vi "Oxford-1820-Main.v.vi"() -> ()   [LabVIEW 2013, in "Mercury iXX.lvlib"]
uses:
  <instrlib>/Mercury iXX/Mercury iXX.lvlib
  <instrlib>/Mercury iXX/Public/Controls/Unit String.ctl
  <instrlib>/Mercury iXX/Public/Libraries/Temperature/Controls/Temperature Device (Read).ctl
  <instrlib>/Mercury iXX/Public/Controls/Manufacturing Data.ctl
  <instrlib>/Mercury iXX/Public/Libraries/Temperature/Controls/Temperature Sensor Type.ctl
  <instrlib>/Mercury iXX/Public/Libraries/Temperature/Controls/Excitation Cluster.ctl
  <instrlib>/Mercury iXX/Public/Libraries/Temperature/Controls/Excitation Type.ctl
  <instrlib>/Mercury iXX/Public/Libraries/Temperature/Controls/Calibration Cluster.ctl
  <instrlib>/Mercury iXX/Public/Libraries/Temperature/Controls/Calibration Interpolation.ctl
  <instrlib>/Mercury iXX/Public/Libraries/Temperature/Controls/Loop Cluster.ctl
  <instrlib>/Mercury iXX/Public/Libraries/Temperature/Controls/Temperature Signals Cluster.ctl
  <instrlib>/Mercury iXX/Public/Libraries/Heater/Controls/Heater Device (Read).ctl
  <instrlib>/Mercury iXX/Public/Libraries/Heater/Controls/Heater Signals Cluster.ctl
  <instrlib>/Mercury iXX/Public/Libraries/Level Meter/Controls/Level Meter (Read).ctl
  <instrlib>/Mercury iXX/Public/Libraries/Level Meter/Controls/Nitrogen Configuration.ctl
  <instrlib>/Mercury iXX/Public/Libraries/Level Meter/Controls/Frequency Configuration.ctl
  <instrlib>/Mercury iXX/Public/Libraries/Level Meter/Controls/Signals.ctl
  <instrlib>/Mercury iXX/Public/Libraries/Level Meter/Controls/Helium Configuration.ctl
  <instrlib>/Mercury iXX/Public/Libraries/Level Meter/Controls/Resistance Configuration.ctl
  <instrlib>/Mercury iXX/Public/Libraries/Level Meter/Controls/Pre-Pulse.ctl
  <instrlib>/Mercury iXX/Public/Libraries/Level Meter/Controls/Pulse.ctl
  <instrlib>/Mercury iXX/Public/Libraries/Auxiliary/Controls/AUX Device (Read).ctl
  <instrlib>/Mercury iXX/Public/Libraries/Auxiliary/Controls/AUX Signals (Read).ctl
  <instrlib>/Mercury iXX/Public/Libraries/Magnet/Controls/Device (Read).ctl
  <instrlib>/Mercury iXX/Public/Libraries/Magnet/Controls/Signals (Read).ctl
  <instrlib>/Mercury iXX/Public/Libraries/Magnet/Controls/Identifier.ctl
  <instrlib>/Mercury iXX/Public/Libraries/Pressure/Controls/Pressure Device (Read).ctl
  <instrlib>/Mercury iXX/Public/Libraries/Pressure/Controls/Pressure Sensor Type.ctl
  <instrlib>/Mercury iXX/Public/Libraries/Pressure/Controls/Calibration Cluster.ctl
  <instrlib>/Mercury iXX/Public/Libraries/Pressure/Controls/Calibration Interpolation.ctl
  <instrlib>/Mercury iXX/Public/Libraries/Pressure/Controls/Loop Cluster.ctl
  <instrlib>/Mercury iXX/Public/Libraries/Pressure/Controls/Pressure Signals Cluster.ctl
  <instrlib>/Mercury iXX/Public/Libraries/Magnet/Controls/PSU Actions.ctl
  <instrlib>/Mercury iXX/Public/Libraries/Magnet/Controls/Switch Heater.ctl
  <instrlib>/Mercury iXX/Public/Controls/Comms Transport Layer.ctl
  <instrlib>/Mercury iXX/Private/Controls/Query Dynamic Reference.ctl
  <instrlib>/Mercury iXX/Public/Controls/Mercury Reference.ctl
  <instrlib>/Mercury iXX/Public/Libraries/Magnet/Open/Open Magnet Device.vi
  <instrlib>/Mercury iXX/Public/Libraries/Magnet/Configuration/Set/PSU Action Status (Set).vi
  <instrlib>/Mercury iXX/Public/Libraries/Magnet/Signals/Read/Current (Read).vi
  <instrlib>/Mercury iXX/Public/Libraries/Magnet/Signals/Read/Persistant Current (Read).vi
  <instrlib>/Mercury iXX/Public/Libraries/Magnet/Signals/Read/Switch Heater Status (Read).vi
  <instrlib>/Mercury iXX/Public/Libraries/Magnet/Signals/Set/Switch Heater No Check (Set).vi
  <instrlib>/Mercury iXX/Public/Libraries/System/Read/Time (Read).vi
  <instrlib>/Mercury iXX/Public/Libraries/Magnet/Signals/Set/Target Field Rate (Set).vi
  <instrlib>/Mercury iXX/Public/Libraries/Magnet/Signals/Set/Target Field (Set).vi
  <instrlib>/Mercury iXX/Public/Libraries/System/Open/Open Device.vi
  <instrlib>/Mercury iXX/Public/Libraries/Control Loop/Configuration/Set/Sweep Mode (Set).vi
  <instrlib>/Mercury iXX/Public/Libraries/System/Open/Open System.vi
  <instrlib>/Mercury iXX/Public/Libraries/System/Read/Catalogue (Read).vi
  <instrlib>/Mercury iXX/Public/Libraries/System/Read/Display Automatic Dimming (Read).vi
  <instrlib>/Mercury iXX/Public/Libraries/System/Read/Display Automatic Dimming Time (Read).vi
  <instrlib>/Mercury iXX/Public/Libraries/System/Read/Display Brightness (Read).vi
  <instrlib>/Mercury iXX/Public/Libraries/System/Read/Date (Read).vi
  <instrlib>/Mercury iXX/Public/Libraries/System/Read/DateTime (Read).vi
  <instrlib>/Mercury iXX/Public/Libraries/System/Read/HVer (Read).vi
  <instrlib>/Mercury iXX/Public/Libraries/System/Read/FVer (Read).vi
  <instrlib>/Mercury iXX/Public/Libraries/System/Read/Serial Number (Read).vi
  <instrlib>/Mercury iXX/Public/Libraries/System/Read/Flash Space (Read).vi
  <instrlib>/Mercury iXX/Public/Libraries/System/Read/Mode (Read).vi
  <instrlib>/Mercury iXX/Public/Libraries/System/Set/DateTime (Set).vi
  <instrlib>/Mercury iXX/Public/Libraries/Temperature/Open/Open Temperature Device.vi
  <instrlib>/Mercury iXX/Public/Libraries/Temperature/Configuration/Read/Serial Number (Read).vi
  <instrlib>/Mercury iXX/Public/Libraries/Temperature/Configuration/Read/Nickname (Read).vi
  <instrlib>/Mercury iXX/Public/Libraries/Temperature/Configuration/Read/Excitation Magnitude (Read).vi
  <instrlib>/Mercury iXX/Public/Libraries/Temperature/Configuration/Read/Temperature Sensor (Read).vi
  <instrlib>/Mercury iXX/Public/Libraries/Temperature/Configuration/Read/Excitation Type (Read).vi
  <instrlib>/Mercury iXX/Public/Libraries/Temperature/Configuration/Read/Calibration Hot Limit (Read).vi
  <instrlib>/Mercury iXX/Public/Libraries/Temperature/Configuration/Read/Calibration Cold Limit (Read).vi
  <instrlib>/Mercury iXX/Public/Libraries/Temperature/Signals/Read/Voltage (Read).vi
  <instrlib>/Mercury iXX/Public/Libraries/Temperature/Signals/Read/Temperature (Read).vi
  <instrlib>/Mercury iXX/Public/Libraries/Temperature/Configuration/Read/Temperature Device (Read).vi
  <instrlib>/Mercury iXX/Public/Libraries/Control Loop/Configuration/Read/Control Loop (Read).vi
  <instrlib>/Mercury iXX/Public/Libraries/Heater/Open/Open Heater Device.vi
  <instrlib>/Mercury iXX/Public/Libraries/Heater/Configuration/Read/Heater Device (Read).vi
  <instrlib>/Mercury iXX/Public/Libraries/Heater/Configuration/Read/Nickname (Read).vi
  <instrlib>/Mercury iXX/Public/Libraries/Heater/Configuration/Read/Serial Number (Read).vi
  <instrlib>/Mercury iXX/Public/Libraries/Heater/Configuration/Read/Voltage Limit (Read).vi
  <instrlib>/Mercury iXX/Public/Libraries/Heater/Configuration/Read/Nominal Resistance (Read).vi
  <instrlib>/Mercury iXX/Public/Libraries/Heater/Configuration/Read/Maximum Power (Read).vi
  <instrlib>/Mercury iXX/Public/Libraries/Heater/Signals/Read/Voltage (Read).vi
  <instrlib>/Mercury iXX/Public/Libraries/Heater/Signals/Read/Power (Read).vi
  <instrlib>/Mercury iXX/Public/Libraries/Heater/Signals/Read/Current (Read).vi
  <instrlib>/Mercury iXX/Public/Libraries/Auxiliary/Open/Open Auxiliary Device.vi
  <instrlib>/Mercury iXX/Public/Libraries/Auxiliary/Configuration/Read/Aux Device (Read).vi
  <instrlib>/Mercury iXX/Public/Libraries/Auxiliary/Configuration/Read/Serial Number (Read).vi
  <instrlib>/Mercury iXX/Public/Libraries/Auxiliary/Configuration/Read/Minimum Gas Flow (Read).vi
  <instrlib>/Mercury iXX/Public/Libraries/Auxiliary/Configuration/Read/Gas Flow Scaling (Read).vi
  <instrlib>/Mercury iXX/Public/Libraries/Auxiliary/Configuration/Read/Temperature Error Sensitivity (Read).vi
  <instrlib>/Mercury iXX/Public/Libraries/Auxiliary/Configuration/Read/Temperature Error Voltage Sensitivity (Read).vi
  <instrlib>/Mercury iXX/Public/Libraries/Auxiliary/Configuration/Read/Valve Gearing (Read).vi
  <instrlib>/Mercury iXX/Public/Libraries/Auxiliary/Configuration/Read/Stepper Speed (Read).vi
  <instrlib>/Mercury iXX/Public/Libraries/Auxiliary/Signals/Read/Position (Read).vi
  <instrlib>/Mercury iXX/Public/Libraries/Auxiliary/Signals/Read/Percent Open (Read).vi
  <instrlib>/Mercury iXX/Public/Libraries/Pressure/Open/Open Pressure Device.vi
  <instrlib>/Mercury iXX/Public/Libraries/Pressure/Configuration/Read/Pressure Device (Read).vi
  <instrlib>/Mercury iXX/Public/Libraries/Pressure/Configuration/Read/Nickname (Read).vi
  <instrlib>/Mercury iXX/Public/Libraries/Pressure/Signals/Read/Current (Read).vi
  <instrlib>/Mercury iXX/Public/Libraries/Pressure/Signals/Read/Voltage (Read).vi
  <instrlib>/Mercury iXX/Public/Libraries/Level Meter/Open/Open Level Meter Device.vi
  <instrlib>/Mercury iXX/Public/Libraries/Level Meter/Configuration/Read/Level Meter Device (Read).vi
  <instrlib>/Mercury iXX/Public/Libraries/Level Meter/Configuration/Read/Serial Number (Read).vi
  <instrlib>/Mercury iXX/Public/Libraries/Level Meter/Configuration/Read/Helium Probe Resistance (Read).vi
  <instrlib>/Mercury iXX/Public/Libraries/Level Meter/Configuration/Read/Helium Pulse Mag (Read).vi
  <instrlib>/Mercury iXX/Public/Libraries/Level Meter/Configuration/Read/Helium Pulse Duration (Read).vi
  <instrlib>/Mercury iXX/Public/Libraries/Level Meter/Configuration/Read/Nitrogen Freq at 100 (Read).vi
  <instrlib>/Mercury iXX/Public/Libraries/Level Meter/Configuration/Read/Nitrogen Pulse Count Period (Read).vi
  <instrlib>/Mercury iXX/Public/Libraries/Level Meter/Signals/Read/Probe Resistance Helium (Read).vi
  <instrlib>/Mercury iXX/Public/Libraries/Level Meter/Signals/Read/Probe Level Helium (Read).vi
  <instrlib>/Mercury iXX/Public/Libraries/Level Meter/Signals/Read/Probe Count Nitrogen (Read).vi
  <instrlib>/Mercury iXX/Public/Libraries/Level Meter/Signals/Read/Probe Level Nitrogen (Read).vi
  <instrlib>/Mercury iXX/Public/Libraries/Magnet/Configuration/Read/Magnet Device (Read).vi
  <instrlib>/Mercury iXX/Public/Libraries/Magnet/Configuration/Read/Serial Number (Read).vi
  <instrlib>/Mercury iXX/Public/Libraries/Magnet/Configuration/Read/Bipolar Output (Read).vi
  <instrlib>/Mercury iXX/Public/Libraries/Magnet/Configuration/Read/Output Configuration (Read).vi
  <instrlib>/Mercury iXX/Public/Libraries/Magnet/Configuration/Read/Current Limit (Read).vi
  <instrlib>/Mercury iXX/Public/Libraries/Magnet/Configuration/Read/Current to Field Factor (Read).vi
  <instrlib>/Mercury iXX/Public/Libraries/Magnet/Configuration/Read/Switch Present (Read).vi
  <instrlib>/Mercury iXX/Public/Libraries/Magnet/Configuration/Read/Software Voltage Limit (Read).vi
  <instrlib>/Mercury iXX/Public/Libraries/Magnet/Signals/Read/Current Rate (Read).vi
  <instrlib>/Mercury iXX/Public/Libraries/Magnet/Configuration/Read/PSU Action Status (Read).vi
  <instrlib>/Mercury iXX/Public/Libraries/Magnet/Signals/Read/Voltage (Read).vi
  <instrlib>/Mercury iXX/Public/Libraries/Magnet/Signals/Read/Field (Read).vi
  <instrlib>/Mercury iXX/Public/Libraries/Magnet/Signals/Read/Target Field Rate (Read).vi
  <instrlib>/Mercury iXX/Public/Libraries/Magnet/Signals/Read/Target Field (Read).vi
  <instrlib>/Mercury iXX/Public/Libraries/Magnet/Signals/Read/Persistant Field (Read).vi
  <instrlib>/Mercury iXX/Public/Libraries/Pressure.lvlib
  <instrlib>/Mercury iXX/Public/Libraries/System.lvlib
  <instrlib>/Mercury iXX/Public/Libraries/Control Loop.lvlib
  <instrlib>/Mercury iXX/Public/Libraries/Heater.lvlib
  <instrlib>/Mercury iXX/Public/Libraries/Temperature.lvlib
  <instrlib>/Mercury iXX/Public/Libraries/Auxiliary.lvlib
  <instrlib>/Mercury iXX/Public/Libraries/Magnet.lvlib
  <instrlib>/Mercury iXX/Public/Libraries/Level Meter.lvlib
  <instrlib>/Mercury iXX/Private/Controls/Command Verbs.ctl
panel:
  out "LPF ON":timestamp
  in  "Tab Control":enum32{"Front Panel", "System Information"}(tab)
  out "Sentinel":bool=TRUE
  in  "OK":bool
  in  "Remote Mode":bool
  out "LPF on (s)":i32=5373
  out "N2 LVL Chart":dbl(slide)=61.3025 scale=0.0..100.0
  out "He LVL Chart":dbl(slide)=52.0833 scale=0.0..100.0
  out "Magnet Field (T)":dbl(knob) caption="Voltage (V)" scale=-20.0..20.0
  in  "Lambda":bool
  out "Magnet Status 2":string
  out "N2 LEVEL":dbl=61.3025 format="%.0f %"
  out "He LEVEL":dbl=52.0833 format="%.0f %"
  out "Switch Time":string="11:11:48"
  out "SWITCH HEATER":bool
  in  "PS Heat":bool
  in  "Clamp":bool
  in  "To Set":bool
  in  "To Zero":bool
  in  "Hold":bool
  out "Magnet Status":string="Clamped"
  out "Target Field Rate (T/min)":dbl=1.0 format="%.5f"
  out "Target Field (T)":dbl format="%#.5f"
  in  "Target Rate (T/min)":dbl=0.1 format="%.5f"
  in  "Target Field (T)":dbl format="%#.5f"
  in  "Send to IPS":bool
  out "Magnet Field (T)":dbl format="%.5f"
  out "Power Supply Field (T)":dbl=0.0001 format="%#.5f"
  out "LPF Temperature":dbl=4.2075 format="%_2f K"
  out "Magnet Temperature":dbl=3.8705 format="%_2f K"
  in  "Fill?":bool=TRUE
  out "Voltage (V)":dbl=-0.0003 format="%.5f"
  out "Current (A)":dbl=0.0006 format="%.5f"
  out "LPF Needle Valve (%)":dbl format="%_6g"
  out "LPF Pressure":dbl format="%_5f mB"
  out "Voltage (V)":dbl(knob)=-0.0003 scale=-10.0..10.0
  out "Current (A)":dbl(knob)=0.0006 scale=-180.0..180.0
  in  "Mercury Functions":T1(tab)=enum."Temperature"
  out "time stamp":timestamp=timestamp(3543841780 s since 1904-01-01)
  out "Free Space":i32=166384 caption="Free Space (KB)"
  out "Set Date Response":string="VALID"
  out "String":string="NORM" caption="User Mode"
  out "Date":string="2016:04:18"
  out "Time":string="11:29:40"
  out "Hardware Version":string="65"
  out "Firmware Version":string="2.2.6.20"
  out "Serial Number":string="154650110"
  out "ITC Devices":string[](array[string])=["DB4.G1:AUX", "DB8.P1:PRES", "MB0.H1:HTR", "MB1.T1:TEMP"]
  out "S/W Version(s)":string[](array[string])=["2.2.6.20\n"]
  out "Serial Number(s)":string[](array[string])=["154650110"]
  out "# of Instruments":i32=1
  out "Automatic Dimming":string="OFF"
  out "Dimming Time":string="5"
  out "Display Brightness":string="100"
  in  "ITC IP Address":string="130.49.180.101"
  out "Excitation Magnitude":dbl=5.0
  out "Sensor Type":string="NTC"
  out "Excitation Type":string="UNIP"
  out "Hot Limit":dbl=1000.0
  out "H Unit":T2="K"
  out "Cold Limit":dbl=1000.0
  out "C Unit":T2="K"
  out "Unit":T2
  out "Voltage":dbl=0.005
  out "V Unit":T2="V"
  out "Temperature":dbl=4.2075
  out "T Unit":T2="K"
  out "Temperature Device Settings":T3={"Manufacturing"={"Hardware Version"="65", "Firmware Version"="2.2", "Serial Number"="154650110"}, "Temperature Sensor Type"="NTC", "Excitation"={"Excitation Type"="UNIP", "Magnitude"="5.00"}, "Calibration"={"Filename"="59543_iTC-lambda.dat", "Interpolation"="LIN", "Scaling Factor"="1", "Offset Factor"="0", "Hot Limit"="1000.00K", "Cold Limit"="1000.00K", "Last Calibration"="", "Reference"="Internal"}, "Control Loop"={"Heater"="", "Auxiliary"="", "Heater Auto"="", "Percentage Heat"="", "Temperature Set Point"="", "PID Auto (from file)"="", "P Value"="", "I Value"="", "D Value"="", "Auto PID Table Filename"="", "Flow Auto"="", "Target Heater Table"="", "Sweep mode"="", "Sweep Table Filename"="", "Percentage Flow"=""}, "Temperature Signals"={"Voltage"="5.0000mV", "Current"="3.9694µA", "Power"="0.0199µW", "Resistance"="1259.6510R", "Temperature"="4.2075K", "Sensitivity"="299.3801R/K", "Reference"="N/A"}, "Nickname"="Mag_AB_MB1", "Status"="0"}
  out "Temp S/N":string="154650110"
  out "T Nickname":string="Mag_AB_MB1"
  out "T Loop Details":T10
  out "Heater Device Settings":T12={"Manufacturing"={"Hardware Version"="65", "Firmware Version"="2.3", "Serial Number"="154650110"}, "Nickname"="MB0.H1", "Voltage Limit"="1", "Nominal Resistance"="10", "Maximum Power"="0.1000", "Heater Signals"={"Voltage"="0.0507V", "Current"="-0.0000A", "Power"="0.0000W"}, "Status"="2"}
  out "Htr C Unit":T2="A"
  out "Htr P Unit":T2="W"
  out "Htr V Unit":T2="V"
  out "Htr Current":dbl=-0.0
  out "Htr Power":dbl
  out "Htr Voltage":dbl=0.0507
  out "Power Unit":T2
  out "Volt Unit":T2
  out "Res Unit":T2
  out "Maximum Power":dbl=0.1
  out "Htr Resistance":dbl=10.0
  out "Htr Voltage Limit":dbl=1.0
  out "Htr S/N":string="154650110"
  out "Htr Nickname":string="MB0.H1"
  out "Pressure Device":T14={"Manufacturing"={"Hardware Version"="3", "Firmware Version"="1.10", "Serial Number"="151150091"}, "Temperature Sensor Type"="RAT", "Calibration"={"Filename"="Lambda pressure control_10V ratiometric.dat", "Interpolation"="LIN", "Scaling Factor"="1", "Offset Factor"="-0.0004", "High Limit"="1000.00K", "Low Limit"="1000.00K", "Last Calibration"=""}, "Control Loop"={"Heater"="None", "Auxiliary"="None", "Heater Auto"="", "Percentage Heat"="", "Pressure Set Point"="", "PID Auto (from file)"="", "P Value"="", "I Value"="", "D Value"="1.0", "Auto PID Table Filename"="", "Flow Auto"="", "Target Heater Table"="", "Sweep mode"="", "Sweep Table Filename"="", "Percentage Flow"=""}, "Pressure Signals"={"Voltage"="-0.0822mV", "Current"="-0.0000A", "Power"="0.0000W", "Pressure"="0.0000mB"}, "Nickname"="Lam_P_DB8", "Status"="0"}
  out "Nickname":string="Lam_P_DB8"
  out "Current":dbl=-0.0
  out "Voltage":dbl=-8.219999999999999e-05
  out "Auxiliary Device Details":T20={"Manufacturing"={"Hardware Version"="65", "Firmware Version"="3.1", "Serial Number"="154650084"}, "Min Flow"=0.0, "Scaling Factor"=50.0, "Temp Err"=9.0, "Temp V Err"=11.0, "Gear"=2, "Speed"=2, "Signals"={"Position"=0.0, "% Open"=0.0, "I0"="ON", "I1"="OFF", "I2"="OFF", "I3"="OFF", "O0"="OFF", "O1"="OFF", "O2"="OFF", "O3"="OFF"}, "Nickname"="DB4.G1", "Status"="0"} {"Signals"."% Open" min=0.0 max=100.0 step=0.1 format="%.4f"; "Signals"."Position" max=20.0 step=1.0 format="%.4f"; "Speed" max=7 step=1; "Gear" max=7 step=1; "Temp V Err" min=0.0 max=20.0 step=0.1; "Temp Err" min=0.0 max=20.0 step=0.1; "Scaling Factor" min=0.0 max=99.0 step=0.1; "Min Flow" min=0.0 max=20.0 step=0.1}
  out "Aux S/N":string="154650084"
  out "Min Flow":dbl caption="Minimum Gas Flow" format="%#.1f"
  out "Scaling Factor":dbl=50.0 caption="Gas Flow Scaling Factor" format="%#.1f"
  out "Temp Err":dbl=9.0 caption="Temperature Error Sensitivity" format="%#.1f"
  out "Temp V Err":dbl=11.0 caption="Temperature Voltage Error Sensitivity" format="%#.1f"
  out "Gear":u32=2 caption="Valve Gearing"
  out "Speed":u32=2 caption="Stepper Speed"
  out "Unit 2":T2
  out "Unit 3":T2
  out "Unit 4":T2
  out "Unit 5":T2
  out "Unit 6":T2
  out "Unit 7":T2
  out "Position":u32
  out "% Open":dbl caption="Percentage Open (%)"
  out "Unit":T2
  out "Unit":T2="%"
  out "time stamp 2":timestamp=timestamp(3543841781 s since 1904-01-01)
  out "Free Space 2":i32=166316 caption="Free Space (KB)"
  out "Set Date Response 2":string="VALID"
  out "String 2":string="NORM" caption="User Mode"
  out "Date 2":string="2016:04:18"
  out "Time 2":string="11:29:45"
  out "Hardware Version 2":string="65"
  out "Firmware Version 2":string="2.2.6.20"
  out "Serial Number 2":string="153350063"
  out "IPS Devices":string[](array[string])=["DB3.L1:LVL", "GRPX:PSU", "GRPY:PSU", "GRPZ:PSU", "MB1.T1:TEMP", "PSU.M1:PSU", "PSU.M2:PSU", "PSU.M3:PSU"]
  out "S/W Version(s) 2":string[](array[string])=["2.2.6.20\n"]
  out "Serial Number(s) 2":string[](array[string])=["153350063"]
  out "# of Instruments 2":i32=1
  out "Automatic Dimming 2":string="OFF"
  out "Dimming Time 2":string="5"
  out "Display Brightness 2":string="100"
  in  "IPS IP Address":string="130.49.180.102"
  out "LVL Device DetailSettings":T22={"Manufacturing"={"Hardware Version"="65", "Firmware Version"="2.2", "Serial Number"="152450013"}, "Nitrogen Configuration"={"Frequency Configuration"={"Freq 0%"=0.0, "Freq 100%"=0.0}, "Pulse Period"=0.0}, "Signals"={"Helium Signals"={"Resistance"=75.5626, "Level"=52.0833}, "Nitrogen Signals"={"Count"=8800.0, "Freq"=487361.0, "Level"=61.3445}}, "Nickname"="DB3.L1", "Status"="0", "Helium Configuration"={"Resistance Configuration"={"Res 0%"=0.0, "Res 100%"=0.0}, "Pre-Pulse"={"Magnitude"=0.0, "Duration"=0.0}, "Pulse"={"Magnitude"=0.0, "Duration"=0.0, "Delay"=0.0}}}
  out "LVL S/N":string="152450013"
  out "LVL P Magnitude":dbl=125.0 caption="Pulse Magnitude (mA)"
  out "LVL P Duration":dbl=5.0 caption="Pulse Duration (s)"
  out "N Freq 100%":dbl=7880.0 caption="Frequency at 100% (Hz)"
  out "N Pulse Period":dbl=1000.0 caption="Pulse Period (ms)"
  out "He Res Config":T27={"Res 0%"=149.0, "Res 100%"=8.0}
  out "He Resistance":dbl=75.5626 caption="Resistance (Ohms)"
  out "He Level":dbl=52.0833 caption="Helium Level (%)"
  out "N Counter":u32 caption="Counter"
  out "N Level":dbl=61.3445 caption="Nitrogen Level (%)"
  out "Excitation Magnitude 2":dbl=5.0
  out "Sensor Type 2":string="NTC"
  out "Excitation Type 2":string="UNIP"
  out "Hot Limit 2":dbl=1000.0
  out "H Unit 2":T2="K"
  out "Cold Limit 2":dbl=1000.0
  out "C Unit 2":T2="K"
  out "Unit 12":T2
  out "Voltage 2":dbl=0.005
  out "V Unit 2":T2="V"
  out "Temperature 2":dbl=3.8706
  out "T Unit 2":T2="K"
  out "Temperature Device Settings 2":T3={"Manufacturing"={"Hardware Version"="65", "Firmware Version"="2.2", "Serial Number"="153350063"}, "Temperature Sensor Type"="NTC", "Excitation"={"Excitation Type"="UNIP", "Magnitude"="5.00"}, "Calibration"={"Filename"="Bob.dat", "Interpolation"="LIN", "Scaling Factor"="1", "Offset Factor"="0", "Hot Limit"="1000.00K", "Cold Limit"="1000.00K", "Last Calibration"="", "Reference"="Internal"}, "Control Loop"={"Heater"="", "Auxiliary"="", "Heater Auto"="", "Percentage Heat"="", "Temperature Set Point"="", "PID Auto (from file)"="", "P Value"="", "I Value"="", "D Value"="", "Auto PID Table Filename"="", "Flow Auto"="", "Target Heater Table"="", "Sweep mode"="", "Sweep Table Filename"="", "Percentage Flow"=""}, "Temperature Signals"={"Voltage"="5.0000mV", "Current"="3.5897µA", "Power"="0.0179µW", "Resistance"="1392.8897R", "Temperature"="3.8706K", "Sensitivity"="359.8580R/K", "Reference"="N/A"}, "Nickname"="MB1.T1", "Status"="0"}
  out "Temp S/N 2":string="153350063"
  out "T Nickname 2":string="MB1.T1"
  out "T Loop Details 2":T10
  out "Magnet Device Details":T30={"Manufacturing"={"Hardware Version"="NOT_FOUND", "Firmware Version"="NOT_FOUND", "Serial Number"="NOT_FOUND"}, "Nickname"="GRPZ", "Bipolar Output"="ON", "String"="PARA", "Current Limit"=174.0, "AtoB"=8.688, "Inductance"=39.406, "Switch Present"="PSU.M1", "Swh Htr Current"=86.0, "SW VLIM"=9.0, "V Trans Time"=1000.0, "Magnet PSU Signals"={"Voltage"=-0.0002, "Current"=0.0002, "Current Rate"=100.0, "Field"=0.0001, "Field Rate"=11.5101, "Persistant Current"=0.0003, "Persistant Field"=0.0, "Target Current"=0.0, "Target Field"=0.0, "Target Current Rate"=8.688, "Target Field Rate"=1.0, "Switch Heater Status (SWHT)"="OFF", "Switch Heater Status (SWHN)"="OFF"}, "PSU Action"="CLMP", "Status"="40000000", "Level Limit"=0.0, "Temperature Limit"=999.0} {"Temperature Limit" format="%#.1f"; "Level Limit" format="%#.1f"; "V Trans Time" format="%#.1f"; "SW VLIM" format="%#.1f"; "Swh Htr Current" format="%#.1f"; "Inductance" format="%#.1f"; "AtoB" format="%#.1f"; "Current Limit" format="%#.1f"}
  out "Mag S/N":string="NOT_FOUND"
  out "Bipolar Output":string="ON"
  out "Out Config":string="PARA" caption="Output Configuration"
  out "Current Limit":dbl=174.0 caption="Current Limit (A)" format="%#.1f"
  out "AtoB":dbl=8.688 caption="Current Field Factor (A/T)" format="%#.1f"
  out "Switch Present":string="PSU.M1"
  out "SW VLIM":dbl=9.0 caption="Software Voltage Limit (V)" format="%#.1f"
  out "Unit 8":T2
  out "Unit 9":T2
  out "Unit 10":T2
  out "Current Rate":dbl=100.0
  out "PSU Act Stat":string="CLMP" caption="PSU Action Status"
  out "Unit 11":T2="A/min"
  in  "Device Identifier":T32="GRPZ"
  # "Voltage (V)"
  # "Magnet (T)"
  # "Current (A)"
  # "He"
  # "N2"
  # "ITC: 101\nIPS: 102\nIPS VR: 67"
  # "ITC: 101\nIPS: 102\nIPS VR: 67"
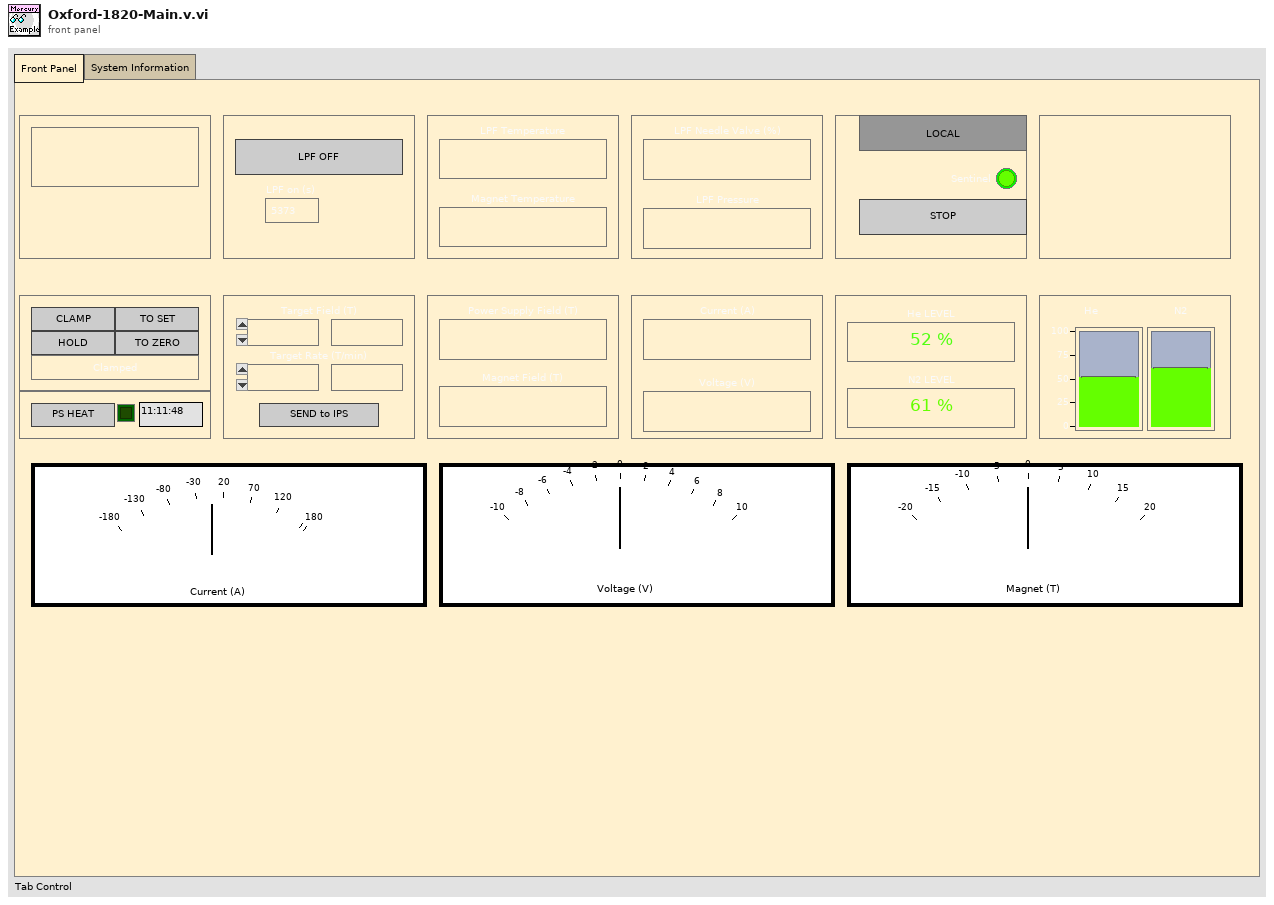
[diagram p1: front panel]
types:
  T1 = enum32{"System: ITC", "Temperature", "Heater", "Pressure", "Auxiliary", "System: IPS", "Level Meter", "Temperature 2", "Magnet"}
  T2 = typedef "Mercury iXX.lvlib/Unit String.ctl" = string
  T3 = typedef "Mercury iXX.lvlib/Temperature.lvlib/Temperature Device (Read).ctl" = cluster{"Manufacturing":T4, "Temperature Sensor Type":T5, "Excitation":T6, "Calibration":T8, "Control Loop":T10, "Temperature Signals":T11, "Nickname":string, "Status":string}
  T4 = typedef "Mercury iXX.lvlib/Manufacturing Data.ctl" = cluster{"Hardware Version":string, "Firmware Version":string, "Serial Number":string}
  T5 = typedef "Mercury iXX.lvlib/Temperature.lvlib/Temperature Sensor Type.ctl" = string
  T6 = typedef "Mercury iXX.lvlib/Temperature.lvlib/Excitation Cluster.ctl" = cluster{"Excitation Type":T7, "Magnitude":string}
  T7 = typedef "Mercury iXX.lvlib/Temperature.lvlib/Excitation Type.ctl" = string
  T8 = typedef "Mercury iXX.lvlib/Temperature.lvlib/Calibration Cluster.ctl" = cluster{"Filename":string, "Interpolation":T9, "Scaling Factor":string, "Offset Factor":string, "Hot Limit":string, "Cold Limit":string, "Last Calibration":string, "Reference":string}
  T9 = typedef "Mercury iXX.lvlib/Temperature.lvlib/Calibration Interpolation.ctl" = string
  T10 = typedef "Mercury iXX.lvlib/Temperature.lvlib/Loop Cluster.ctl" = cluster{"Heater":string, "Auxiliary":string, "Heater Auto":string, "Percentage Heat":string, "Temperature Set Point":string, "PID Auto (from file)":string, "P Value":string, "I Value":string, "D Value":string, "Auto PID Table Filename":string, "Flow Auto":string, "Target Heater Table":string, "Sweep mode":string, "Sweep Table Filename":string, "Percentage Flow":string}
  T11 = typedef "Mercury iXX.lvlib/Temperature.lvlib/Temperature Signals Cluster.ctl" = cluster{"Voltage":string, "Current":string, "Power":string, "Resistance":string, "Temperature":string, "Sensitivity":string, "Reference":string}
  T12 = typedef "Mercury iXX.lvlib/Heater.lvlib/Heater Device (Read).ctl" = cluster{"Manufacturing":T4, "Nickname":string, "Voltage Limit":string, "Nominal Resistance":string, "Maximum Power":string, "Heater Signals":T13, "Status":string}
  T13 = typedef "Mercury iXX.lvlib/Heater.lvlib/Heater Signals Cluster.ctl" = cluster{"Voltage":string, "Current":string, "Power":string}
  T14 = typedef "Mercury iXX.lvlib/Pressure.lvlib/Pressure Device (Read).ctl" = cluster{"Manufacturing":T4, "Temperature Sensor Type":T15, "Calibration":T16, "Control Loop":T18, "Pressure Signals":T19, "Nickname":string, "Status":string}
  T15 = typedef "Mercury iXX.lvlib/Pressure.lvlib/Pressure Sensor Type.ctl" = string
  T16 = typedef "Mercury iXX.lvlib/Pressure.lvlib/Calibration Cluster.ctl" = cluster{"Filename":string, "Interpolation":T17, "Scaling Factor":string, "Offset Factor":string, "High Limit":string, "Low Limit":string, "Last Calibration":string}
  T17 = typedef "Mercury iXX.lvlib/Pressure.lvlib/Calibration Interpolation.ctl" = string
  T18 = typedef "Mercury iXX.lvlib/Pressure.lvlib/Loop Cluster.ctl" = cluster{"Heater":string, "Auxiliary":string, "Heater Auto":string, "Percentage Heat":string, "Pressure Set Point":string, "PID Auto (from file)":string, "P Value":string, "I Value":string, "D Value":string, "Auto PID Table Filename":string, "Flow Auto":string, "Target Heater Table":string, "Sweep mode":string, "Sweep Table Filename":string, "Percentage Flow":string}
  T19 = typedef "Mercury iXX.lvlib/Pressure.lvlib/Pressure Signals Cluster.ctl" = cluster{"Voltage":string, "Current":string, "Power":string, "Pressure":string}
  T20 = typedef "Mercury iXX.lvlib/Auxiliary.lvlib/AUX Device (Read).ctl" = cluster{"Manufacturing":T4, "Min Flow":dbl, "Scaling Factor":dbl, "Temp Err":dbl, "Temp V Err":dbl, "Gear":u32, "Speed":u32, "Signals":T21, "Nickname":string, "Status":string}
  T21 = typedef "Mercury iXX.lvlib/Auxiliary.lvlib/AUX Signals (Read).ctl" = cluster{"Position":dbl, "% Open":dbl, "I0":string, "I1":string, "I2":string, "I3":string, "O0":string, "O1":string, "O2":string, "O3":string}
  T22 = typedef "Mercury iXX.lvlib/Level Meter.lvlib/Level Meter (Read).ctl" = cluster{"Manufacturing":T4, "Nitrogen Configuration":T23, "Signals":T25, "Nickname":string, "Status":string, "Helium Configuration":T26}
  T23 = typedef "Mercury iXX.lvlib/Level Meter.lvlib/Nitrogen Configuration.ctl" = cluster{"Frequency Configuration":T24, "Pulse Period":dbl}
  T24 = typedef "Mercury iXX.lvlib/Level Meter.lvlib/Frequency Configuration.ctl" = cluster{"Freq 0%":dbl, "Freq 100%":dbl}
  T25 = typedef "Mercury iXX.lvlib/Level Meter.lvlib/Signals.ctl" = cluster{"Helium Signals":cluster{"Resistance":dbl, "Level":dbl}, "Nitrogen Signals":cluster{"Count":dbl, "Freq":dbl, "Level":dbl}}
  T26 = typedef "Mercury iXX.lvlib/Level Meter.lvlib/Helium Configuration.ctl" = cluster{"Resistance Configuration":T27, "Pre-Pulse":T28, "Pulse":T29}
  T27 = typedef "Mercury iXX.lvlib/Level Meter.lvlib/Resistance Configuration.ctl" = cluster{"Res 0%":dbl, "Res 100%":dbl}
  T28 = typedef "Mercury iXX.lvlib/Level Meter.lvlib/Pre-Pulse.ctl" = cluster{"Magnitude":dbl, "Duration":dbl}
  T29 = typedef "Mercury iXX.lvlib/Level Meter.lvlib/Pulse.ctl" = cluster{"Magnitude":dbl, "Duration":dbl, "Delay":dbl}
  T30 = typedef "Mercury iXX.lvlib/Magnet.lvlib/Device (Read).ctl" = cluster{"Manufacturing":T4, "Nickname":string, "Bipolar Output":string, "String":string, "Current Limit":dbl, "AtoB":dbl, "Inductance":dbl, "Switch Present":string, "Swh Htr Current":dbl, "SW VLIM":dbl, "V Trans Time":dbl, "Magnet PSU Signals":T31, "PSU Action":string, "Status":string, "Level Limit":dbl, "Temperature Limit":dbl}
  T31 = typedef "Mercury iXX.lvlib/Magnet.lvlib/Signals (Read).ctl" = cluster{"Voltage":dbl, "Current":dbl, "Current Rate":dbl, "Field":dbl, "Field Rate":dbl, "Persistant Current":dbl, "Persistant Field":dbl, "Target Current":dbl, "Target Field":dbl, "Target Current Rate":dbl, "Target Field Rate":dbl, "Switch Heater Status (SWHT)":string, "Switch Heater Status (SWHN)":string}
  T32 = typedef "Mercury iXX.lvlib/Magnet.lvlib/Identifier.ctl" = string
  T33 = cluster{"Hold":bool, "Clamp":bool, "To Set":bool, "To Zero":bool, "Send to IPS":bool, "PS Heat":bool, "Lambda":bool}
  T34 = typedef "Mercury iXX.lvlib/Magnet.lvlib/PSU Actions.ctl" = string
  T35 = typedef "Mercury iXX.lvlib/Magnet.lvlib/Switch Heater.ctl" = string
  T36 = typedef "Mercury iXX.lvlib/Command Verbs.ctl" = string
  T37 = enum32{"invalid app kind", "Development System", "Run Time System", "Student Edition", "Embedded LabVIEW", "Evaluation", "Custom"}
  T38 = enum32{"Invalid", "Standard", "Closed", "Hidden", "Minimized", "Maximized"}
  T39 = cluster{"Persistant Field":dbl, "Field":dbl, "Target Field":dbl, "Target Field Rate":dbl, "Voltage":dbl, "Current":dbl}
  T40 = typedef "Mercury iXX.lvlib/Comms Transport Layer.ctl" = enum16{"Ethernet TCP/IP", "USB", "ISOBus - RS-232", "GPIB"}
  T41 = typedef "Mercury iXX.lvlib/Query Dynamic Reference.ctl" = refnum<vi>
  T42 = typedef "Mercury iXX.lvlib/Mercury Reference.ctl" = cluster{"Comms":refnum<visa-resource-name>, "Device ID":string[], "Comms Layer":T40, "Command":string, "Query reference":T41}
  T43 = cluster{"Core":cluster{"Current VI Reference":refnum<vi>, "Close Panel on Exit?":bool}, "Mercury ITC Ref":cluster{"Comms":refnum<visa-resource-name>, "Device ID":string[], "Comms Layer":T40, "Command":string, "Query reference":T41}, "Mercury IPS Ref":T42, "sentinel":bool}
  T44 = typedef "Mercury iXX.lvlib/Response String.ctl" = string
  T45 = cluster{"Target Field (T)":dbl, "Target Field Rate (T/min)":dbl}
  T46 = cluster{"Comms":refnum<visa-resource-name>, "Device ID":string[], "Comms Layer":T40, "Command":string, "Query reference":T41}
  T47 = cluster{"Current VI Reference":refnum<vi>, "Close Panel on Exit?":bool}
  T48 = typedef "Mercury iXX.lvlib/System.lvlib/User Mode.ctl" = string
  T49 = typedef "Mercury iXX.lvlib/Magnet.lvlib/Output Configuration.ctl" = string
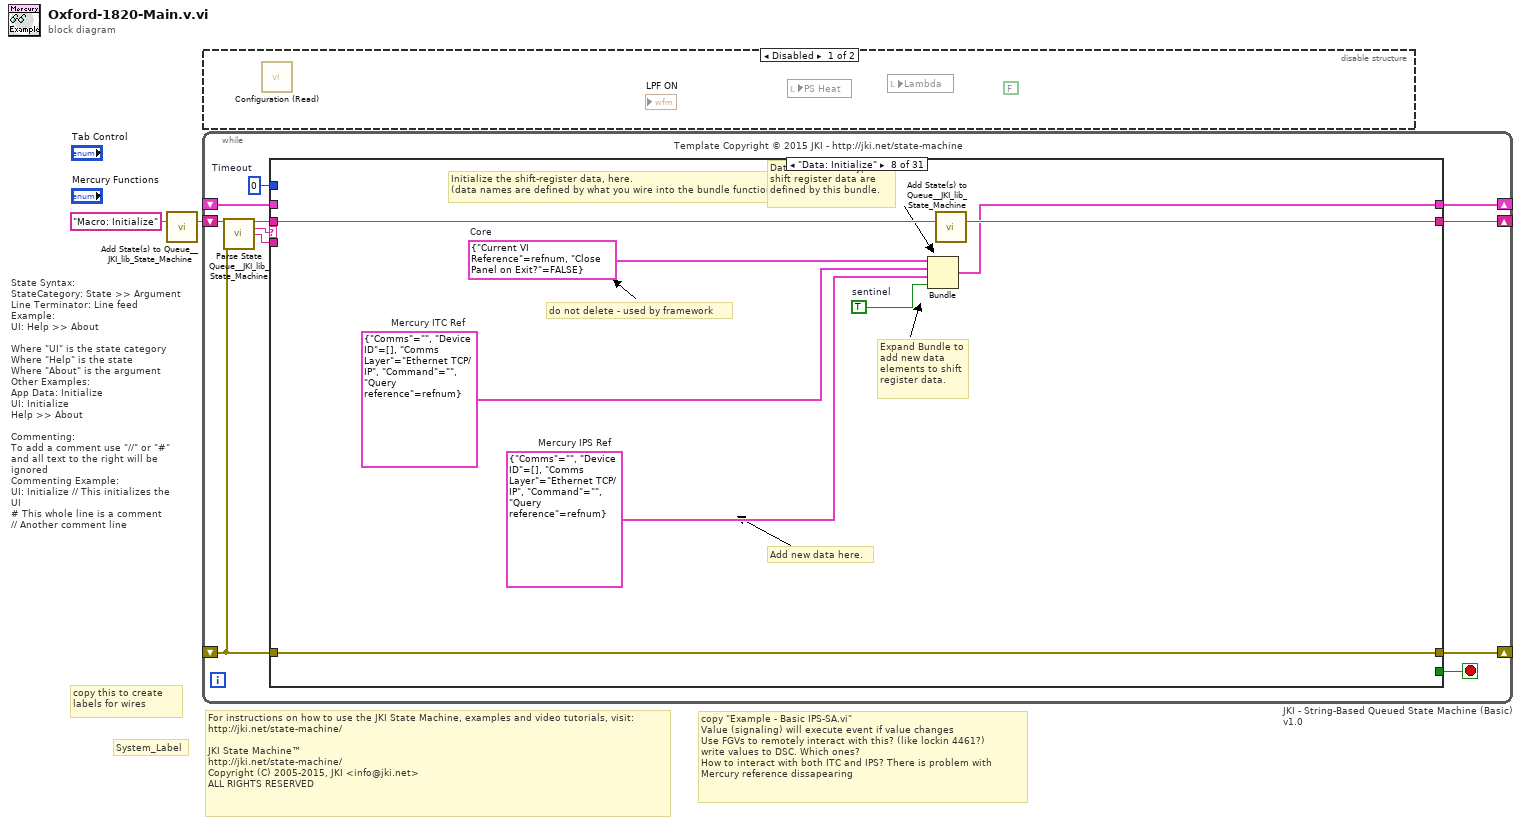
[diagram p0: block diagram]
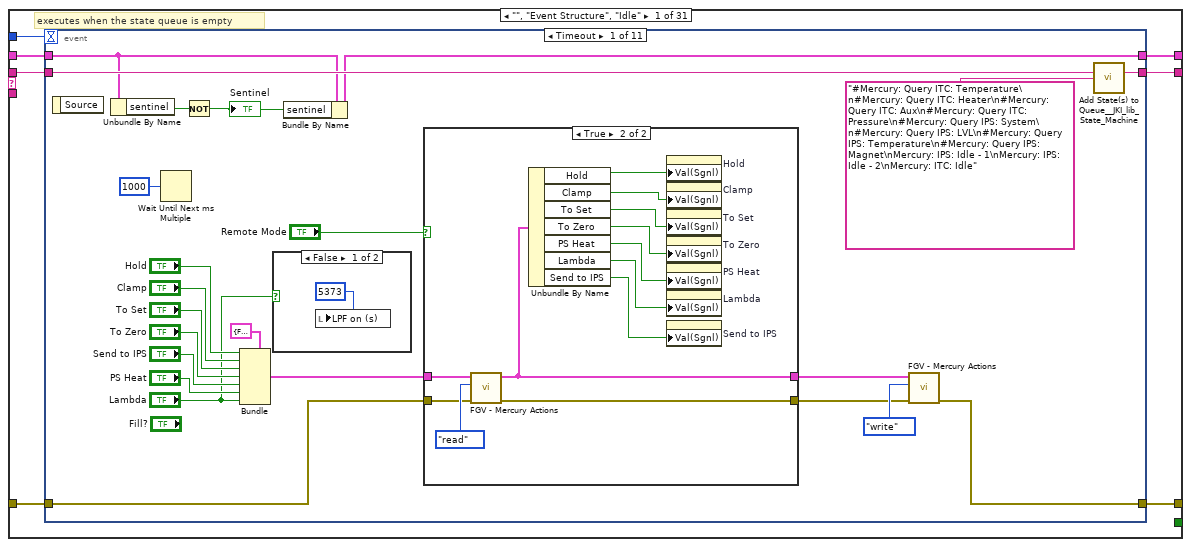
[diagram p3: hidden frame]
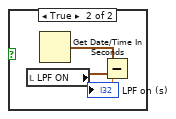
[diagram p4: hidden frame]
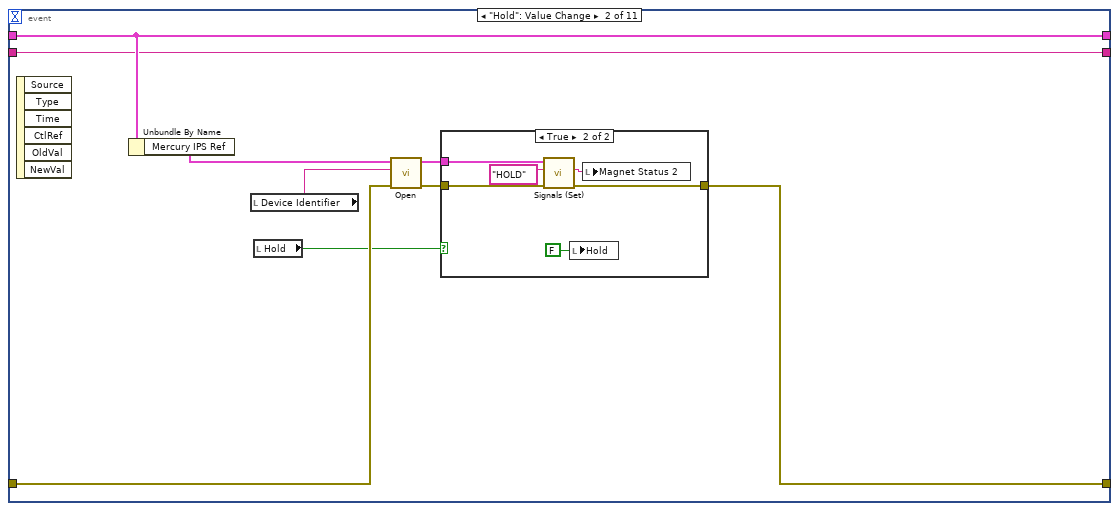
[diagram p6: hidden frame]
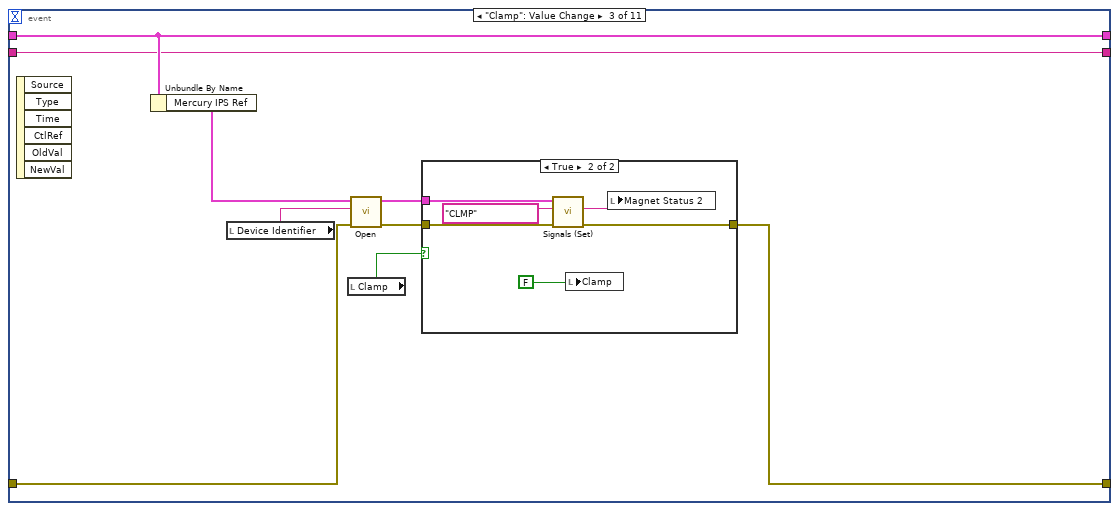
[diagram p8: hidden frame]
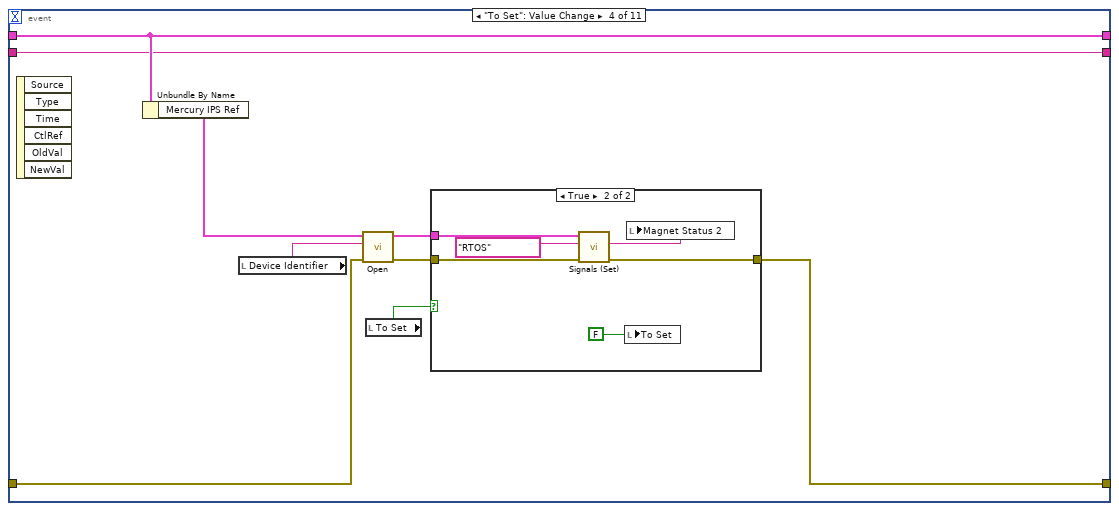
[diagram p10: hidden frame]
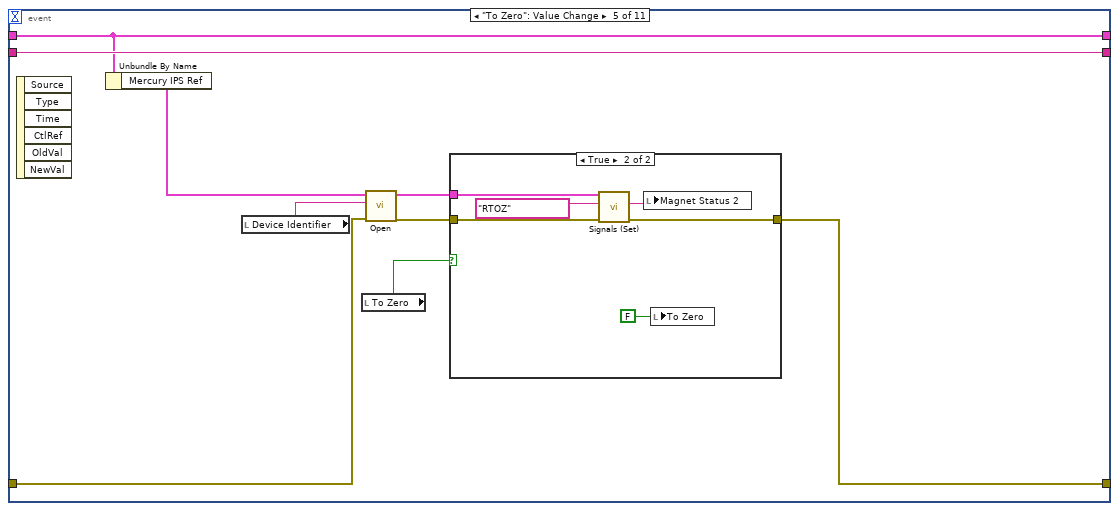
[diagram p12: hidden frame]
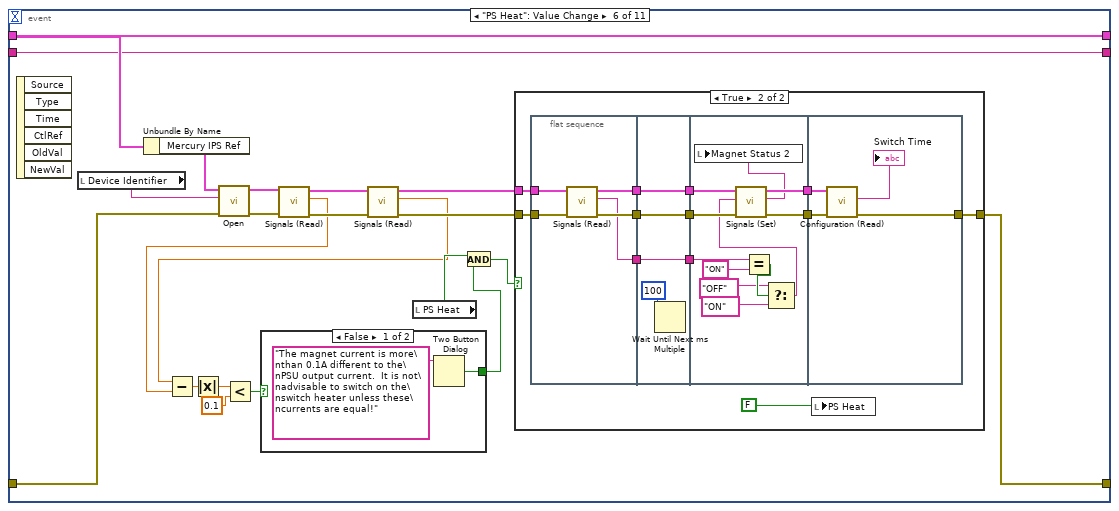
[diagram p14: hidden frame]
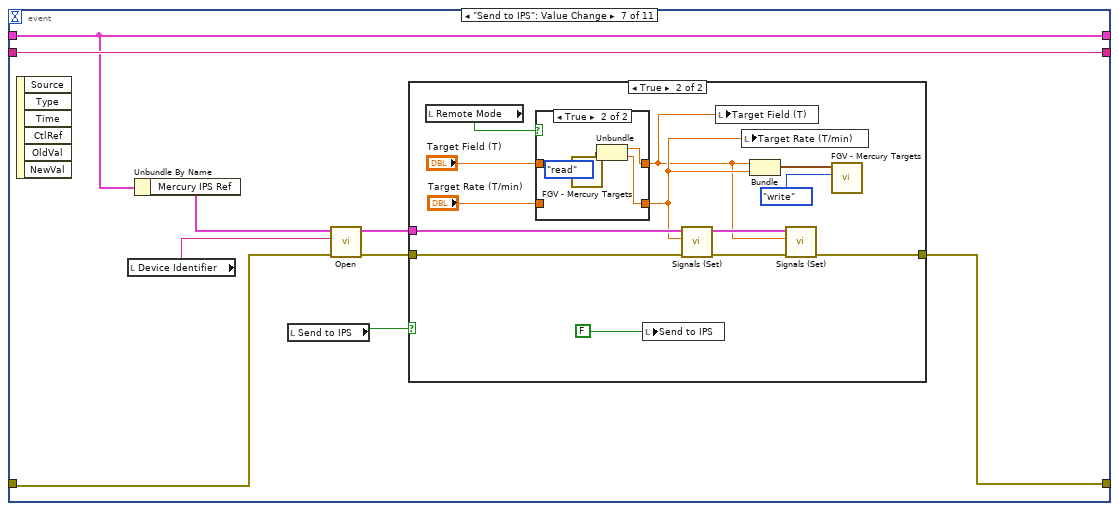
[diagram p17: hidden frame]
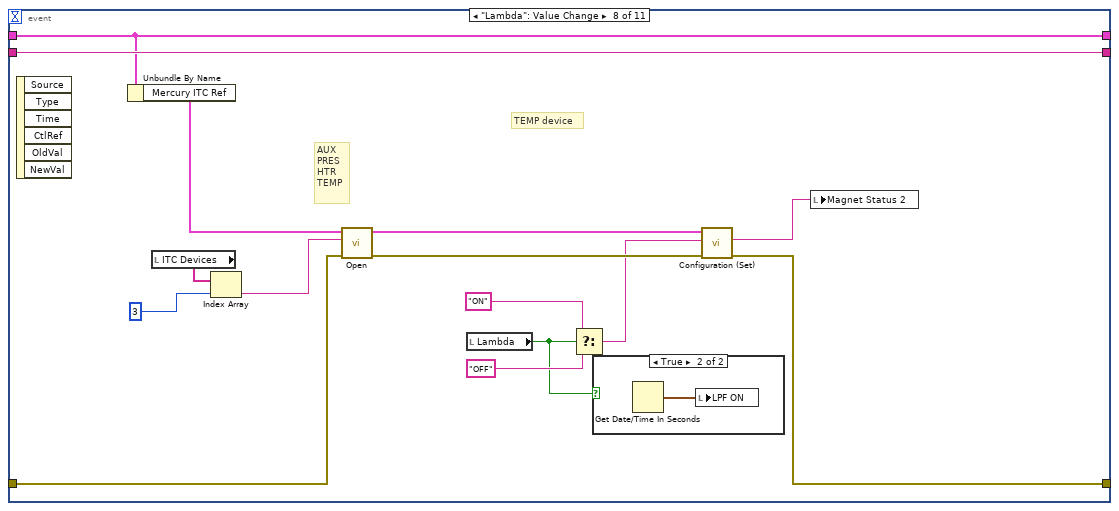
[diagram p20: hidden frame]
diagram:
  # "copy \"Example - Basic IPS-SA.vi\"\nValue (signaling) will execute event if value changes\nUse FGVs to remotely interact with this? (like lockin 4461?)\nwrite values to DSC. Which ones?\nHow to interact with both ITC and IPS? There is problem with \nMercury reference dissapearing"
  # "For instructions on how to use the JKI State Machine, examples and video tutorials, visit:\nhttp://jki.net/state-machine/\n\nJKI State Machine™\nhttp://jki.net/state-machine/\nCopyright (C) 2005-2015, JKI <info@jki.net>\nALL RIGHTS RESERVED"
  # "State Syntax:\nStateCategory: State >> Argument\nLine Terminator: Line feed\nExample:\nUI: Help >> About\n\nWhere \"UI\" is the state category\nWhere \"Help\" is the state\nWhere \"About\" is the argument\nOther Examples:\nApp Data: Initialize\nUI: Initialize\nHelp >> About\n\nCommenting:\nTo add a comment use \"//\" or \"#\" and all text to the right will be ignored\nCommenting Example:\nUI: Initialize // This initializes the UI\n# This whole line is a comment\n// Another comment line"
  # "copy this to create labels for wires"
  # "System_Label"
  n1 = call <vilib>:"Add State(s) to Queue__JKI_lib_State_Machine.vi"("State(s) in (\"\")"="Macro: Initialize") -> ("States Out"=w2:string)  [unwired: 14 in]
  n2 = while "JKI - String-Based Queued State Machine (Basic) v1.0" {
    shift-right: [w6] -> _
    shift-left: _ -> [w5]
    shift-right: [w9] -> _
    shift-left: _ -> [w3]
    shift-right: [w8] -> _
    shift-left: w2 -> [w10]
    stop <- w7 stop-if-true
    w4 = 0  # Timeout
    # "Template Copyright © 2015 JKI - http://jki.net/state-machine"
    n3 = call <vilib>:"Parse State Queue__JKI_lib_State_Machine.vi"("State Queue"=w10, "Error In (no error)"=w3) -> ("Remaining States"=w12:string, "Current State"=w13:string, "Arguments"=w11:string)  [unwired: 11 in]
    n4 = case shown="\"Data: Initialize\"" w13 {
      selector: w13 -> [_ _ w263 _ _ _ _ _ _ _ _ _ _ _ _ _ _ _ _ _ _ _ _ _ _ _ _ _ _ _ _]
      tunnel: w12 -> [w20 w262 w267 w285 w291 w296 w300 w308 w314 w318 w323 w329 w340 w366 w371 w386 w390 w413 w457 w503 w545 w592 w613 w658 w699 w746 w787 w824 w878 w917 w921]
      tunnel: w11 -> [_ _ _ _ _ _ _ _ _ _ _ w324 w334 _ _ _ _ _ _ _ _ _ _ _ _ _ _ _ _ _ _]
      tunnel: w5 -> [w16 w259 w265 w276 w288 w294 w297 _ w309 w315 w321 w327 w336 w363 w369 w384 w387 w408 w455 w502 w509 w552 w599 w656 w698 w745 w786 w823 w877 w916 w920]
      tunnel: [w14 w260 w269 w282 errorcluster {"status"=FALSE, "code"=0, "source"=""} ("error out") w293 w298 w305 w310 w316 w320 w325 w337 w364 w368 w372 w388 w392 w417 w464 w506 w555 w600 w620 w665 w704 w753 w789 w854 w890 w919] -> w9
      tunnel: w3 -> [w15 w260 w268 w282 w287 w293 w298 w305 w311 w316 w320 w326 w338 w364 w368 w374 w388 w400 w419 w465 w512 w554 w594 w622 w667 w701 w748 w822 w855 w891 w919]
      tunnel: [w19 w261 w266 w284 w290 w295 w299 w307 w313 w317 w322 w328 w339 w365 w370 w385 w389 w412 w456 w504 w546 w593 w614 w657 w700 w747 w788 w825 w879 w918 w922] -> w8
      tunnel: [_ _ _ _ _ TRUE _ _ _ _ _ _ _ _ _ _ _ _ _ _ _ _ _ _ _ _ _ _ _ _ _] -> w7
      tunnel: [w18 w259 w265 w283 w288 w294 w297 w306 w309 w315 w321 w327 w336 w363 w369 w384 w387 w407 w455 w502 w509 w552 w599 w656 w698 w745 w786 w823 w877 w916 w920] -> w6
      tunnel: w4 -> [w17 _ _ _ _ _ _ _ _ _ _ _ _ _ _ _ _ _ _ _ _ _ _ _ _ _ _ _ _ _ _]
      frame "", "Event Structure", "Idle" {
        # "executes when the state queue is empty"
        n5 = event shown="[0] Timeout" {
          selector: _ -> [_ _ _ _ _ _ _ _ _ _ _]
          dyn-events: _ -> [_ _ _ _ _ _ _ _ _ _ _]
          timeout: w17 -> [_ _ _ _ _ _ _ _ _ _ _]
          tunnel: w20 -> [w43 w69 w85 w100 w117 w137 w195 w230 w234 w252 w258]
          tunnel: [w42 w69 w85 w100 w117 w137 w195 w230 w234 w251 w257] -> w19
          tunnel: [w37 w70 w86 w101 w116 w138 w191 w228 w235 w249 w255] -> w18
          tunnel: w16 -> [w38 w70 w86 w101 w116 w138 w191 w228 w235 w249 w255]
          tunnel: w15 -> [w28 w66 w80 w95 w111 w129 w194 w222 w233 w250 w256]
          tunnel: [w31 w68 w84 w102 w118 w136 w192 w221 w233 w250 w256] -> w14
          event Timeout {
            n6 = event-data() -> ()  [unwired: 1 in, 1 out]
            n7 = Unbundle By Name(w38) -> ("sentinel"=w40:bool)
            n8 = Wait Until Next ms Multiple(millisecond multiple=u32 1000) -> ()  [unwired: 1 out]
            n9 = Not(x=w40) -> (.not. x?=w39:bool)
            "Sentinel" <- w39
            n10 = Bundle(cluster=T33 {"Hold"=FALSE, "Clamp"=FALSE, "To Set"=FALSE, "To Zero"=FALSE, "Send to IPS"=FALSE, "PS Heat"=FALSE, "Lambda"=FALSE}, "Hold"="Hold", "Clamp"="Clamp", "To Set"="To Set", "To Zero"="To Zero", "Send to IPS"="Send to IPS", "PS Heat"="PS Heat", "Lambda"="Lambda") -> (w27:T33)
            n11 = case shown="False" "Lambda" {
              frame False {
                n12 = local write "LPF on (s)"(5373 ("LPF on (s)")) -> ()
              }
              frame True {
                n13 = local read "LPF ON"() -> (w47:timestamp)
                n14 = Get Date/Time In Seconds() -> (seconds since 1Jan1904=w46:timestamp)
                n15 = Subtract(x=w46, y=w47) -> (x-y=→"LPF on (s)":dbl)
              }
            }
            n16 = Bundle By Name(cluster=w38, "sentinel"=w39) -> (w37:T43)
            n17 = case shown="True" "Remote Mode" {
              tunnel: [w48 w53] -> w29
              tunnel: w28 -> [w48 w52]
              tunnel: w27 -> [w49 w51]
              tunnel: [w49 w50] -> w26
              frame False {
              }
              frame True {
                n18 = call "FGV - Mercury Actions.vi"("error in"=w52, "Function"=enum16{"write", "read"}."read", "mercury actions"=w51) -> ("error out"=w53:errorcluster, "Mercury actions"=w50:T33)  [unwired: 3 in]
                n19 = Unbundle By Name(w50) -> ("Hold"=w61:bool, "Clamp"=w60:bool, "To Set"=w59:bool, "To Zero"=w58:bool, "PS Heat"=w57:bool, "Lambda"=w56:bool, "Send to IPS"=w55:bool)
                n20 = property on="Hold" class="Bool (strict)"("Val(Sgnl)"=w61) -> ()  [unwired: 2 in, 2 out]
                n21 = property on="Clamp" class="Bool (strict)"("Val(Sgnl)"=w60) -> ()  [unwired: 2 in, 2 out]
                n22 = property on="To Set" class="Bool (strict)"("Val(Sgnl)"=w59) -> ()  [unwired: 2 in, 2 out]
                n23 = property on="To Zero" class="Bool (strict)"("Val(Sgnl)"=w58) -> ()  [unwired: 2 in, 2 out]
                n24 = property on="PS Heat" class="Bool (strict)"("Val(Sgnl)"=w57) -> ()  [unwired: 2 in, 2 out]
                n25 = property on="Lambda" class="Bool (strict)"("Val(Sgnl)"=w56) -> ()  [unwired: 2 in, 2 out]
                n26 = property on="Send to IPS" class="Bool (strict)"("Val(Sgnl)"=w55) -> ()  [unwired: 2 in, 2 out]
              }
            }
            n27 = call "FGV - Mercury Actions.vi"("error in"=w29, "Function"=enum16{"write", "read"}."write", "mercury actions"=w26) -> ("error out"=w31:errorcluster)  [unwired: 3 in, 1 out]
            n28 = call <vilib>:"Add State(s) to Queue__JKI_lib_State_Machine.vi"("State(s) in (\"\")"=w43, "State(s) at Back (\"\")"="#Mercury: Query ITC: Temperature\n#Mercury: Query ITC: Heater\n#Mercury: Query ITC: Aux\n#Mercury: Query ITC: Pressure\n#Mercury: Query IPS: System\n#Mercury: Query IPS: LVL\n#Mercury: Query IPS: Temperature\n#Mercury: Query IPS: Magnet\nMercury: IPS: Idle - 1\nMercury: IPS: Idle - 2\nMercury: ITC: Idle" ("State(s) at Back (\"\")")) -> ("States Out"=w42:string)  [unwired: 13 in]
          }
          event "Hold": Value Change {
            n29 = event-data() -> ()  [unwired: 1 in, 6 out]
            n30 = Unbundle By Name(w70) -> ("Mercury IPS Ref"=w64:T42)
            n31 = local read "Device Identifier"() -> (w65:T32)
            n32 = local read "Hold"() -> (w62:bool)
            n33 = call-poly <instrlib>:"Open.vi"("error in (no error)"=w66, "Device Identifier"=w65, "Mercury Reference In"=w64) -> ("error out"=w67:errorcluster, "Mercury Reference Out"=w63:T42)  [unwired: 7 out]
            n34 = case shown="True" w62 {
              tunnel: [w71 w76] -> w68
              tunnel: w67 -> [w71 w75]
              tunnel: w63 -> [_ w74]
              frame False {
              }
              frame True {
                n35 = call-poly <instrlib>:"Signals (Set).vi"("error in"=w75, "PSU Act Stat"=T34 "HOLD", "Mercury Reference In"=w74) -> ("error out"=w76:errorcluster, "Response"=w72:T44)  [unwired: 1 in, 6 out]
                n36 = local write "Hold"(FALSE ("Hold")) -> ()
                n37 = local write "Magnet Status 2"(w72) -> ()
              }
            }
          }
          event "Clamp": Value Change {
            n38 = event-data() -> ()  [unwired: 1 in, 6 out]
            n39 = Unbundle By Name(w86) -> ("Mercury IPS Ref"=w79:T42)
            n40 = local read "Device Identifier"() -> (w83:T32)
            n41 = local read "Clamp"() -> (w78:bool)
            n42 = call-poly <instrlib>:"Open.vi"("error in (no error)"=w80, "Device Identifier"=w83, "Mercury Reference In"=w79) -> ("error out"=w82:errorcluster, "Mercury Reference Out"=w81:T42)  [unwired: 7 out]
            n43 = case shown="True" w78 {
              tunnel: [w87 w92] -> w84
              tunnel: w82 -> [w87 w90]
              tunnel: w81 -> [_ w89]
              frame False {
              }
              frame True {
                n44 = call-poly <instrlib>:"Signals (Set).vi"("error in"=w90, "PSU Act Stat"=T34 "CLMP", "Mercury Reference In"=w89) -> ("error out"=w92:errorcluster, "Response"=w91:T44)  [unwired: 1 in, 6 out]
                n45 = local write "Clamp"(FALSE) -> ()
                n46 = local write "Magnet Status 2"(w91) -> ()
              }
            }
          }
          event "To Set": Value Change {
            n47 = event-data() -> ()  [unwired: 1 in, 6 out]
            n48 = Unbundle By Name(w101) -> ("Mercury IPS Ref"=w97:T42)
            n49 = local read "Device Identifier"() -> (w96:T32)
            n50 = call-poly <instrlib>:"Open.vi"("error in (no error)"=w95, "Device Identifier"=w96, "Mercury Reference In"=w97) -> ("error out"=w98:errorcluster, "Mercury Reference Out"=w99:T42)  [unwired: 7 out]
            n51 = local read "To Set"() -> (w94:bool)
            n52 = case shown="True" w94 {
              tunnel: [w103 w108] -> w102
              tunnel: w99 -> [_ w106]
              tunnel: w98 -> [w103 w105]
              frame False {
              }
              frame True {
                n53 = call-poly <instrlib>:"Signals (Set).vi"("error in"=w105, "PSU Act Stat"=T34 "RTOS", "Mercury Reference In"=w106) -> ("error out"=w108:errorcluster, "Response"=w107:T44)  [unwired: 1 in, 6 out]
                n54 = local write "To Set"(FALSE) -> ()
                n55 = local write "Magnet Status 2"(w107) -> ()
              }
            }
          }
          event "To Zero": Value Change {
            n56 = event-data() -> ()  [unwired: 1 in, 6 out]
            n57 = Unbundle By Name(w116) -> ("Mercury IPS Ref"=w113:T42)
            n58 = local read "Device Identifier"() -> (w112:T32)
            n59 = local read "To Zero"() -> (w110:bool)
            n60 = call-poly <instrlib>:"Open.vi"("error in (no error)"=w111, "Device Identifier"=w112, "Mercury Reference In"=w113) -> ("error out"=w114:errorcluster, "Mercury Reference Out"=w115:T42)  [unwired: 7 out]
            n61 = case shown="True" w110 {
              tunnel: [w119 w124] -> w118
              tunnel: w115 -> [_ w122]
              tunnel: w114 -> [w119 w121]
              frame False {
              }
              frame True {
                n62 = call-poly <instrlib>:"Signals (Set).vi"("error in"=w121, "PSU Act Stat"=T34 "RTOZ", "Mercury Reference In"=w122) -> ("error out"=w124:errorcluster, "Response"=w123:T44)  [unwired: 1 in, 6 out]
                n63 = local write "Magnet Status 2"(w123) -> ()
                n64 = local write "To Zero"(FALSE) -> ()
              }
            }
          }
          event "PS Heat": Value Change {
            n65 = event-data() -> ()  [unwired: 1 in, 6 out]
            n66 = local read "Device Identifier"() -> (w130:T32)
            n67 = Unbundle By Name(w138) -> ("Mercury IPS Ref"=w134:T42)
            n68 = call-poly <instrlib>:"Open.vi"("error in (no error)"=w129, "Device Identifier"=w130, "Mercury Reference In"=w134) -> ("error out"=w126:errorcluster, "Mercury Reference Out"=w127:T42)  [unwired: 7 out]
            n69 = call-poly <instrlib>:"Signals (Read).vi"("error in"=w126, "Mercury Reference In"=w127) -> ("error out"=w140:errorcluster, "Current"=w135:dbl, "Mercury Reference Out"=w139:T42)  [unwired: 1 in, 6 out]
            n70 = call-poly <instrlib>:"Signals (Read).vi"("error in"=w140, "Mercury Reference In"=w139) -> ("error out"=w141:errorcluster, "Persistant Current"=w128:dbl, "Mercury Reference Out"=w142:T42)  [unwired: 1 in, 6 out]
            n71 = Subtract(x=w128, y=w135) -> (x-y=w143:dbl)
            n72 = Absolute Value(x=w143) -> (abs(x)=w144:dbl)
            n73 = Less?(x=w144, y=0.1) -> (x < y?=w146:bool)
            n74 = case shown="False" w146 {
              selector: w146 -> [_ w149]
              tunnel: [w148 w149] -> w132
              frame False {
                n75 = Two Button Dialog(message="The magnet current is more\nthan 0.1A different to the\nPSU output current.  It is not\nadvisable to switch on the\nswitch heater unless these\ncurrents are equal!") -> (T button?=w148:bool)  [unwired: 2 out]
              }
              frame True {
              }
            }
            n76 = local read "PS Heat"() -> (w133:bool)
            n77 = And(x=w133, y=w132) -> (x .and. y?=w131:bool)
            n78 = case shown="True" w131 {
              tunnel: w142 -> [_ w154]
              tunnel: w141 -> [w150 w153]
              tunnel: [w150 w152] -> w136
              frame False {
              }
              frame True {
                n79 = flat-sequence {
                  tunnel: [w165] -> w162
                  tunnel: [w164] -> w161
                  tunnel: [w163] -> w160
                  tunnel: w154 -> [w167]
                  tunnel: w153 -> [w166]
                  tunnel: w162 -> [w170]
                  tunnel: w161 -> [w169]
                  tunnel: [w170] -> w159
                  tunnel: [w169] -> w158
                  tunnel: [w168] -> w157
                  tunnel: w160 -> [w168]
                  tunnel: w159 -> [w181]
                  tunnel: w158 -> [w182]
                  tunnel: w157 -> [w179]
                  tunnel: [w176] -> w156
                  tunnel: [w177] -> w155
                  tunnel: w156 -> [w186]
                  tunnel: w155 -> [w185]
                  tunnel: [w184] -> w152
                  frame #0 {
                    n80 = call-poly <instrlib>:"Signals (Read).vi"("error in"=w166, "Mercury Reference In"=w167) -> ("error out"=w165:errorcluster, "Switch Heater Status"=w163:string, "Mercury Reference Out"=w164:T42)  [unwired: 1 in, 6 out]
                  }
                  frame #1 {
                    n81 = Wait Until Next ms Multiple(millisecond multiple=u32 100) -> ()  [unwired: 1 out]
                  }
                  frame #2 {
                    n82 = Equal?(x=w179, y="ON") -> (x = y?=w178:bool)
                    n83 = Select(t=T35 "OFF" ("Set Switch Heater"), s=w178, f=T35 "ON" ("Set Switch Heater")) -> (s? t:f=w173:T35)
                    n84 = call-poly <instrlib>:"Signals (Set).vi"("error in"=w181, "Set Switch Heater"=w173, "Mercury Reference In"=w182) -> ("error out"=w177:errorcluster, "Response"=w172:T44, "Mercury Reference Out"=w176:T42)  [unwired: 1 in, 5 out]
                    n85 = local write "Magnet Status 2"(w172) -> ()
                  }
                  frame #3 {
                    n86 = call-poly <instrlib>:"Configuration (Read).vi"("error in"=w185, "Mercury Reference In"=w186) -> ("error out"=w184:errorcluster, "Time"=→"Switch Time":string)  [unwired: 1 in, 7 out]
                  }
                }
                n87 = local write "PS Heat"(FALSE) -> ()
              }
            }
          }
          event "Send to IPS": Value Change {
            n88 = event-data() -> ()  [unwired: 1 in, 6 out]
            n89 = local read "Device Identifier"() -> (w190:T32)
            n90 = Unbundle By Name(w191) -> ("Mercury IPS Ref"=w189:T42)
            n91 = local read "Send to IPS"() -> (w187:bool)
            n92 = call-poly <instrlib>:"Open.vi"("error in (no error)"=w194, "Device Identifier"=w190, "Mercury Reference In"=w189) -> ("error out"=w193:errorcluster, "Mercury Reference Out"=w188:T42)  [unwired: 7 out]
            n93 = case shown="True" w187 {
              tunnel: w193 -> [w196 w209]
              tunnel: [w196 w207] -> w192
              tunnel: w188 -> [_ w206]
              frame False {
              }
              frame True {
                n94 = local read "Remote Mode"() -> (w203:bool)
                n95 = case shown="True" w203 {
                  tunnel: "Target Field (T)" -> [w211 _]
                  tunnel: "Target Rate (T/min)" -> [w210 _]
                  tunnel: [w211 w213] -> w197
                  tunnel: [w210 w212] -> w198
                  frame False {
                  }
                  frame True {
                    n96 = call "FGV - Mercury Targets.vi"("Function"=enum16{"write", "read"}."read") -> ("Mercury Targets"=w214:T45)  [unwired: 5 in, 1 out]
                    n97 = Unbundle(w214) -> ("Target Field (T)"=w213:dbl, "Target Field Rate (T/min)"=w212:dbl)
                  }
                }
                n98 = local write "Send to IPS"(FALSE) -> ()
                n99 = call-poly <instrlib>:"Signals (Set).vi"("error in"=w209, "Target Field Rate"=w198, "Mercury Reference In"=w206) -> ("error out"=w208:errorcluster, "Mercury Reference Out"=w205:T42)  [unwired: 2 in, 5 out]
                n100 = local write "Target Field (T)"(w197) -> ()
                n101 = local write "Target Rate (T/min)"(w198) -> ()
                n102 = Bundle("Target Field (T)"=w197, "Target Field Rate (T/min)"=w198) -> (w200:T45)  [unwired: 1 in]
                n103 = call-poly <instrlib>:"Signals (Set).vi"("error in"=w208, "Target Field"=w197, "Mercury Reference In"=w205) -> ("error out"=w207:errorcluster)  [unwired: 2 in, 6 out]
                n104 = call "FGV - Mercury Targets.vi"("Function"=enum16{"write", "read"}."write", "Mercury Targets"=w200) -> ()  [unwired: 4 in, 2 out]
              }
            }
          }
          event "Lambda": Value Change {
            # "AUX\nPRES\nHTR\nTEMP"
            # "TEMP device"
            n105 = event-data() -> ()  [unwired: 1 in, 6 out]
            n106 = Unbundle By Name(w228) -> ("Mercury ITC Ref"=w227:T46)
            n107 = local read "ITC Devices"() -> (w229:string[])
            n108 = Index Array(array=w229, index=3) -> (element=w226:string)
            n109 = call-poly <instrlib>:"Open.vi"("error in (no error)"=w222, "Device Identifier"=w226, "Mercury Reference In"=w227) -> ("error out"=w223:errorcluster, "Mercury Reference Out"=w224:T42)  [unwired: 1 in, 6 out]
            n110 = local read "Lambda"() -> (w218:bool)
            n111 = Select(t="ON" ("Sweep Mode"), s=w218, f="OFF" ("Sweep Mode")) -> (s? t:f=w220:string)
            n112 = case shown="True" w218 {
              frame False {
                n113 = local write "LPF ON"(timestamp(0 s since 1904-01-01) ("LPF ON")) -> ()
              }
              frame True {
                n114 = Get Date/Time In Seconds() -> (seconds since 1Jan1904=w232:timestamp)
                n115 = local write "LPF ON"(w232) -> ()
              }
            }
            n116 = call-poly <instrlib>:"Configuration (Set).vi"("error in"=w223, "Sweep Mode"=w220, "Mercury Reference In"=w224) -> ("error out"=w221:errorcluster, "Response"=w219:T44)  [unwired: 5 in, 2 out]
            n117 = local write "Magnet Status 2"(w219) -> ()
          }
          event "Fill?": Value Change {
            n118 = event-data() -> ()  [unwired: 1 in, 6 out]
            n119 = disable-structure shown="Disabled" {
              frame Disabled {
                w246 = FALSE  # fast/slow
                n120 = Unbundle By Name() -> ()  [unwired: 1 in, 1 out]
                n121 = local read "IPS Devices"() -> (w236:string[])
                n122 = Index Array(array=w236, index=0) -> ()  [unwired: 1 out]
                n123 = call-poly <instrlib>:"Open.vi"() -> ()  [unwired: 3 in, 9 out]
                n124 = Select(t=0.0 ("Temperature setpoint"), s=w246, f=1.0 ("Temperature setpoint")) -> (s? t:f=w241:dbl)
                n125 = call <instrlib>:"Build SCPI Command.vi"("Noun(s)"=":HEL:PULS:SLOW", "Verb"=T36 "SET:") -> ("error out"=w244:errorcluster, "SCPI Message(s)"=w238:string[], "Mercury Reference Out"=w245:T42, "Mercury Reference In"=w247:T42)  [unwired: 6 in]
                n126 = call <instrlib>:"Set (DBL).vi"("error in"=w244, "Command Value (Dbl)"=w241, "SCPI Message(s)"=w238, "Mercury Reference In"=w245) -> ()  [unwired: 4 in, 4 out]
              }
              frame Enabled {
              }
            }
          }
          event "OK": Value Change {
            # "Exit Button Value Change (pressed) Event\n(this executes Macro: Exit to terminate the VI)"
            n127 = event-data() -> ()  [unwired: 1 in, 1 out]
            n128 = call <vilib>:"Add State(s) to Queue__JKI_lib_State_Machine.vi"("State(s) in Front (\"\")"="Macro: Exit", "State(s) in (\"\")"=w252) -> ("States Out"=w251:string)  [unwired: 13 in]
          }
          event Panel Close? {
            # "Discard the event because we'll close the front panel ourselves in Macro: Exit"
            # "Close Panel button (pressed) Event\n(this executes Macro: Exit to terminate the VI)"
            n129 = event-data() -> ()  [unwired: 1 in, 1 out]
            n130 = call <vilib>:"Add State(s) to Queue__JKI_lib_State_Machine.vi"("State(s) in Front (\"\")"="Macro: Exit", "State(s) in (\"\")"=w258) -> ("States Out"=w257:string)  [unwired: 13 in]
            n131 = event-data("Discard?"=TRUE) -> ()  [unwired: 1 in, 1 out]
          }
        }
      }
      frame "---------- Core ----------" {
        # "Do not put any code in this frame.\n(it is a separator no-op)"
        n132 = call <vilib>:"Add State(s) to Queue__JKI_lib_State_Machine.vi"("State(s) in (\"\")"=w262) -> ("States Out"=w261:string)  [unwired: 14 in]
      }
      frame Default {
        w272 = 42 items=["No error", "Argument error", "Memory is full", "Out of zone", "End of file", "File already open", "Generic file I/O error", "File not found", "File permission error", "Disk is full", "Duplicate path", "Too many files open", "System feature not enabled", "Resource file not found", "Cannot add resource", "Resource not found", "Image not found", "Image memory error", "Pen does not exist", "Config type invalid", "Config token not found", "Config parse error", "Config memory error", "Bad external code format", "Bad external code offset", "External code not present", "Null window", "Destroy window error", "Null menu", "Print aborted", "Bad print record", "Print driver error", "Windows error during printing", "Memory error during printing", "Print dialog error", "Generic print error", "Invalid device refnum", "Device not found", "Device parameter error", "Device unit error", "Cannot open device", "Device call aborted", "Generic error", "Cancelled by user", "Object ID too low", "Object ID too high", "Object not in heap", "Unknown heap", "Unknown object (invalid DefProc)", "Unknown object (DefProc not in table)", "Message out of range", "Invalid (null) method", "Unknown message", "Manager call not supported", "Bad address", "Network operation in progress", "Network operation timed out", "Connection is busy", "Network attribute not supported", "Network error", "Address in use", "System out of memory", "Connection aborted", "Connection refused", "Not connected", "Already connected", "Connection closed", "Initialization error (interapplication manager)", "Bad occurrence", "Wait on unbound occurrence handler", "Occurrence queue overflow", "Datalog type conflict", "Unused", "Unrecognized type (interapplication manager)", "Memory corrupt", "Failed to make temporary DLL", "Old CIN version", "Drag socket not found", "Failed to load drop-object", "Failed to register OLE object", "Failed to release OLE object", "Format specifier type mismatch", "Unknown format specifier", "Too few format specifiers", "Too many format specifiers", "Scan failed", "Newer CIN version", "Error converting to variant", "Runtime menu error", "Password tampered", "Variant attribute not found", "Incompatible variant data type", "Event data is not available", "Event Store is not present", "Occurrence is not found", "Event Queue is not created", "Event info is not available", "Refnum passed is NULL", "Error retrieving Class GUID", "Error retrieving CoClass GUID", "Error retrieving TypeLib GUID.", "Bad built application magic bytes.", "Specific driver is different from the specific driver associated with the Logical Name.", "There is no session opened to the class driver.", "Max Error", "MAX - Error with config objects", "MAX - Error loading configuration", "MAX - Group not supported"]
        # "Current State"
        # "Do not delete, rename, or modify this frame.\n(this is used to capture unhandled states and typos)"
        # "Handle mistyped state name (developer tool)"
        n133 = Format Into String(format string="Software Exception: Unhandled State \"%s\"." ("message"), error in=w268, w263) -> (resulting string=w271:string, error out=w270:errorcluster)  [unwired: 1 in]
        n134 = call <vilib>:"Error Cluster From Error Code.vi"("show call chain? (False)"=TRUE, "error in (no error)"=w270, "error message (\"\")"=w271, "error code (0)"=w272) -> ("error out"=w269:errorcluster)  [unwired: 5 in]
        n135 = call <vilib>:"Add State(s) to Queue__JKI_lib_State_Machine.vi"("State(s) in (\"\")"=w267) -> ("States Out"=w266:string)  [unwired: 14 in]
      }
      frame "Initialize Core Data" {
        # "Do not delete, rename, or modify this frame.\n(this is used to determine panel behavior on exit)"
        # "originally closed?"
        # "exe?"
        # "If panel starts closed or is an EXE, then close it when we exit"
        n136 = property class="VI"() -> ("Front Panel.Open"=w281:bool)  [unwired: 2 in, 2 out]
        n137 = property class="App"() -> ("App.Kind"=w280:T37)  [unwired: 2 in, 2 out]
        n138 = control-ref of="Current VI Reference"() -> (w274:refnum<vi>)
        n139 = Not(x=w281) -> (.not. x?=w278:bool)
        n140 = Equal?(x=w280, y=T37."Run Time System" ("Application:Kind")) -> (x = y?=w277:bool)
        n141 = Or(x=w278, y=w277) -> (x .or. y?=w275:bool)
        n142 = Bundle By Name(cluster=w276, "Core.Current VI Reference"=w274, "Core.Close Panel on Exit?"=w275) -> (w283:T43)
        n143 = call <vilib>:"Add State(s) to Queue__JKI_lib_State_Machine.vi"("State(s) in (\"\")"=w285) -> ("States Out"=w284:string)  [unwired: 14 in]
      }
      frame "Error Handler" {
        # "Unhandled Error -- Display it"
        # "Handle any errors here.\nYou can also output any states to clean-up after errors occur"
        # "Clear error"
        n144 = call <vilib>:"General Error Handler.vi"("error in (no error)"=w287) -> ()  [unwired: 10 in, 5 out]
        n145 = call <vilib>:"Add State(s) to Queue__JKI_lib_State_Machine.vi"("State(s) in Front (\"\")"="/* Post Error States", "State(s) in (\"\")"=w291) -> ("States Out"=w290:string)  [unwired: 13 in]
      }
      frame "Exit" {
        # "Do not put any code in this frame.\n(No errors that occur here will be handled.)"
        n146 = call <vilib>:"Add State(s) to Queue__JKI_lib_State_Machine.vi"("State(s) in (\"\")"=w296) -> ("States Out"=w295:string)  [unwired: 14 in]
      }
      frame "---------- Data ----------" {
        # "Do not put any code in this frame.\n(It is a separator no-op. You can make a copy of this frame to create a new Data frame)"
        n147 = call <vilib>:"Add State(s) to Queue__JKI_lib_State_Machine.vi"("State(s) in (\"\")"=w300) -> ("States Out"=w299:string)  [unwired: 14 in]
      }
      frame "Data: Initialize" {
        w301 = TRUE  # sentinel
        w302 = T42 {"Comms"="", "Device ID"=[], "Comms Layer"=enum."Ethernet TCP/IP", "Command"="", "Query reference"=refnum}  # Mercury IPS Ref
        w303 = T46 {"Comms"="", "Device ID"=[], "Comms Layer"=enum."Ethernet TCP/IP", "Command"="", "Query reference"=refnum}  # Mercury ITC Ref
        w304 = T47 {"Current VI Reference"=refnum, "Close Panel on Exit?"=FALSE}  # Core
        # "do not delete - used by framework"
        # "Expand Bundle to add new data elements to shift register data."
        # "Add new data here."
        # "Data names and types of shift register data are defined by this bundle."
        # "Initialize the shift-register data, here.\n(data names are defined by what you wire into the bundle function)"
        n148 = Bundle("Core"=w304, "Mercury ITC Ref"=w303, "Mercury IPS Ref"=w302, "sentinel"=w301) -> (w306:T43)  [unwired: 1 in]
        n149 = call <vilib>:"Add State(s) to Queue__JKI_lib_State_Machine.vi"("State(s) in (\"\")"=w308) -> ("States Out"=w307:string)  [unwired: 14 in]
      }
      frame "Data: Cleanup" {
        # "Cleanup any data and references, here.\n(this is called automatically, by the Macro: Exit)"
        n150 = Unbundle By Name(w309) -> ("Core.Current VI Reference"=w312:refnum<vi>)
        n151 = Close Reference(reference=w312, error in (no error)=w311) -> (error out=w310:errorcluster)
        n152 = call <vilib>:"Add State(s) to Queue__JKI_lib_State_Machine.vi"("State(s) in (\"\")"=w314) -> ("States Out"=w313:string)  [unwired: 14 in]
      }
      frame "---------- UI ----------" {
        # "Do not put any code in this frame.\n(It is a separator no-op. You can make a copy of this frame to create a new UI frame)"
        n153 = call <vilib>:"Add State(s) to Queue__JKI_lib_State_Machine.vi"("State(s) in (\"\")"=w318) -> ("States Out"=w317:string)  [unwired: 14 in]
      }
      frame "UI: Initialize" {
        # "Initialize the User Interface, here.\n(this is called automatically, by the Macro: Init)"
        n154 = call <vilib>:"Add State(s) to Queue__JKI_lib_State_Machine.vi"("State(s) in (\"\")"=w323) -> ("States Out"=w322:string)  [unwired: 14 in]
        "Magnet Status 2" <- "" ("Magnet Status 2")
      }
      frame "UI: Cursor Set" {
        # "Argument"
        # "Set and Unset Cursor Busy.\n(Usage: \"UI: Cursor Set >> Busy|Idle\")"
        n155 = case shown="\"Idle\", Default" w324 {
          tunnel: w326 -> [w331 w333]
          tunnel: [w330 w332] -> w325
          frame "Idle", Default {
            n156 = call <vilib>:"Unset Busy.vi"("error in (no error)"=w331) -> ("error out"=w330:errorcluster)  [unwired: 10 in]
          }
          frame "Busy" {
            n157 = call <vilib>:"Set Busy.vi"("error in (no error)"=w333) -> ("error out"=w332:errorcluster)  [unwired: 9 in, 1 out]
          }
        }
        n158 = call <vilib>:"Add State(s) to Queue__JKI_lib_State_Machine.vi"("State(s) in (\"\")"=w329) -> ("States Out"=w328:string)  [unwired: 14 in]
      }
      frame "UI: Front Panel State" {
        # "Argument"
        # "Set Front Panel Open or Closed\n(Usage: \"UI: Front Panel State >> Open|Close\")"
        n159 = Unbundle By Name(w336) -> ("Core.Current VI Reference"=w335:refnum<vi>)
        n160 = case shown="\"Open\", Default" w334 {
          tunnel: w338 -> [w344 w357]
          tunnel: [w346 w358] -> w337
          tunnel: w335 -> [w345 w355]
          frame "Open", Default {
            n161 = property class="VI"(reference=w345, error in=w344) -> (reference out=w342:refnum<vi>, error out=w343:errorcluster, "Front Panel.Open"=w341:bool)
            n162 = case shown="True" w341 {
              tunnel: [w349 w352] -> w346
              tunnel: w343 -> [w348 w352]
              tunnel: w342 -> [w347 _]
              frame False {
                n163 = invoke class="VI" method="FP.Open"(reference=w347, error in=w348, "Activate"=TRUE, "State"=T38."Standard") -> (error out=w349:errorcluster)  [unwired: 1 in, 4 out]
              }
              frame True {
              }
            }
          }
          frame "Close" {
            n164 = property class="VI"(reference=w355, error in=w357) -> (reference out=w354:refnum<vi>, error out=w356:errorcluster, "Front Panel.Open"=w353:bool)
            n165 = case shown="True" w353 {
              tunnel: [w359 w362] -> w358
              tunnel: w356 -> [w359 w361]
              tunnel: w354 -> [_ w360]
              frame False {
              }
              frame True {
                n166 = invoke class="VI" method="FP.Close"(reference=w360, error in=w361) -> (error out=w362:errorcluster)  [unwired: 1 in, 2 out]
              }
            }
          }
        }
        n167 = call <vilib>:"Add State(s) to Queue__JKI_lib_State_Machine.vi"("State(s) in (\"\")"=w340) -> ("States Out"=w339:string)  [unwired: 14 in]
      }
      frame "---------- Macro ----------" {
        # "Do not put any code in this frame.\n(It is a separator no-op. You can make a copy of this frame to create a new Macro frame)"
        n168 = call <vilib>:"Add State(s) to Queue__JKI_lib_State_Machine.vi"("State(s) in (\"\")"=w366) -> ("States Out"=w365:string)  [unwired: 14 in]
      }
      frame "Macro: Initialize" {
        w367 = "Data: Initialize\nInitialize Core Data\nUI: Initialize\nUI: Front Panel State >> Open\nMercury: Initialize"  # Data: Initialize Initialize Core Data UI: Initialize UI: Front Panel State >> Open Mercury: Initialize
        # "Initialization Macro\n(This is called once, when the VI starts)"
        n169 = call <vilib>:"Add State(s) to Queue__JKI_lib_State_Machine.vi"("State(s) in Front (\"\")"=w367, "State(s) in (\"\")"=w371) -> ("States Out"=w370:string)  [unwired: 13 in]
      }
      frame "Macro: Exit" {
        # "Exit Macro\n(This is called once, when the VI exits)"
        n170 = Unbundle By Name(w384) -> ("Core.Close Panel on Exit?"=w383:bool, "Mercury ITC Ref"=w376:T46, "Mercury IPS Ref"=w375:T42)
        n171 = call <instrlib>:"Close.vi"("error in (no error)"=w374, "Mercury Reference"=w375) -> ("error out"=w373:errorcluster)  [unwired: 9 out]
        n172 = call <instrlib>:"Close.vi"("error in (no error)"=w373, "Mercury Reference"=w376) -> ("error out"=w377:errorcluster)  [unwired: 9 out]
        n173 = call <vilib>:"Simple Error Handler.vi"("error in (no error)"=w377) -> ("error out"=w372:errorcluster)  [unwired: 1 in, 7 out]
        n174 = Select(t="UI: Front Panel State >> Close", s=w383, f="") -> (s? t:f=w380:string)
        n175 = call <vilib>:"Add State(s) to Queue__JKI_lib_State_Machine.vi"("State(s) in (\"\")"=w380, "State(s) at Back (\"\")"="Data: Cleanup\nExit") -> ("States Out"=w378:string)  [unwired: 13 in]
        n176 = call <vilib>:"Add State(s) to Queue__JKI_lib_State_Machine.vi"("State(s) in Front (\"\")"=w378, "State(s) in (\"\")"=w386) -> ("States Out"=w385:string)  [unwired: 13 in]
      }
      frame "---------- New Category ----------" {
        n177 = call <vilib>:"Add State(s) to Queue__JKI_lib_State_Machine.vi"("State(s) in (\"\")"=w390) -> ("States Out"=w389:string)  [unwired: 14 in]
      }
      frame "Mercury: Initialize" {
        w399 = Comms_Transport_Layer."Ethernet TCP/IP" ("Comms Layer")
        n178 = call-poly <instrlib>:"Open.vi"("Clear Previous Connections (False)"=TRUE ("Clear Previous Connections (True)"), "ID Query (True)"=TRUE, "IP Address"="ITC IP Address", "error in (no error)"=w400, "Comms Layer"=w399) -> ("error out"=w393:errorcluster, "# of Instruments"=→"# of Instruments":i32, "Serial Number(s)"=→"Serial Number(s)":string[], "Mercury Reference Out"=w394:T42, "S/W Version(s)"=→"S/W Version(s)":string[])  [unwired: 2 in]
        n179 = call-poly <instrlib>:"Open.vi"("Clear Previous Connections (False)"=FALSE ("Clear Previous Connections (True)"), "ID Query (True)"=TRUE, "IP Address"="IPS IP Address", "error in (no error)"=w393, "Comms Layer"=w399) -> ("error out"=w392:errorcluster, "# of Instruments"=→"# of Instruments 2":i32, "Serial Number(s)"=→"Serial Number(s) 2":string[], "Mercury Reference Out"=w391:T42, "S/W Version(s)"=→"S/W Version(s) 2":string[])  [unwired: 2 in]
        n180 = Bundle By Name(cluster=w408, "Mercury ITC Ref"=w394, "Mercury IPS Ref"=w391) -> (w407:T43)
        n181 = call <vilib>:"Add State(s) to Queue__JKI_lib_State_Machine.vi"("State(s) in (\"\")"=w413, "State(s) at Back (\"\")"="Mercury: Query ITC: System\nMercury: Query IPS: System\nMercury: Query ITC: Temperature\nMercury: Query ITC: Heater\nMercury: Query ITC: Aux\nMercury: Query ITC: Pressure\nMercury: Query IPS: LVL\nMercury: Query IPS: Temperature\nMercury: Query IPS: Magnet" ("State(s) at Back (\"\")")) -> ("States Out"=w412:string)  [unwired: 13 in]
      }
      frame "Mercury: Query ITC: System" {
        n182 = Unbundle By Name(w455) -> ("Mercury ITC Ref"=w415:T46)
        n183 = call-poly <instrlib>:"Configuration (Read).vi"("error in"=w419, "Mercury Reference In"=w415) -> ("error out"=w451:errorcluster, "Devices"=→"ITC Devices":string[], "Mercury Reference Out"=w452:T42)  [unwired: 1 in, 6 out]
        n184 = call-poly <instrlib>:"Configuration (Read).vi"("error in"=w451, "Mercury Reference In"=w452) -> ("error out"=w444:errorcluster, "Automatic Dimming"=→"Automatic Dimming":string, "Mercury Reference Out"=w445:T42)  [unwired: 1 in, 6 out]
        n185 = call-poly <instrlib>:"Configuration (Read).vi"("error in"=w444, "Mercury Reference In"=w445) -> ("error out"=w447:errorcluster, "Dimming Time"=→"Dimming Time":string, "Mercury Reference Out"=w446:T42)  [unwired: 1 in, 6 out]
        n186 = call-poly <instrlib>:"Configuration (Read).vi"("error in"=w447, "Mercury Reference In"=w446) -> ("error out"=w453:errorcluster, "Display Brightness"=→"Display Brightness":string, "Mercury Reference Out"=w454:T42)  [unwired: 1 in, 6 out]
        n187 = call-poly <instrlib>:"Configuration (Read).vi"("error in"=w453, "Mercury Reference In"=w454) -> ("error out"=w438:errorcluster, "Date"=→"Date":string, "Mercury Reference Out"=w437:T42)  [unwired: 1 in, 6 out]
        n188 = call-poly <instrlib>:"Configuration (Read).vi"("error in"=w438, "Mercury Reference In"=w437) -> ("error out"=w440:errorcluster, "Time"=→"Time":string, "Mercury Reference Out"=w439:T42)  [unwired: 1 in, 6 out]
        n189 = call-poly <instrlib>:"Configuration (Read).vi"("error in"=w440, "Mercury Reference In"=w439) -> ("error out"=w418:errorcluster, "time stamp"=→"time stamp":timestamp, "Mercury Reference Out"=w416:T42)  [unwired: 1 in, 6 out]
        n190 = call-poly <instrlib>:"Configuration (Read).vi"("error in"=w418, "Mercury Reference In"=w416) -> ("error out"=w436:errorcluster, "Hardware Version"=→"Hardware Version":string, "Mercury Reference Out"=w435:T42)  [unwired: 1 in, 6 out]
        n191 = call-poly <instrlib>:"Configuration (Read).vi"("error in"=w436, "Mercury Reference In"=w435) -> ("error out"=w434:errorcluster, "Firmware Version"=→"Firmware Version":string, "Mercury Reference Out"=w433:T42)  [unwired: 1 in, 6 out]
        n192 = call-poly <instrlib>:"Configuration (Read).vi"("error in"=w434, "Mercury Reference In"=w433) -> ("error out"=w421:errorcluster, "Serial Number"=→"Serial Number":string, "Mercury Reference Out"=w420:T42)  [unwired: 1 in, 6 out]
        n193 = call-poly <instrlib>:"Configuration (Read).vi"("error in"=w421, "Mercury Reference In"=w420) -> ("error out"=w427:errorcluster, "Free Space"=→"Free Space":i32, "Mercury Reference Out"=w426:T42)  [unwired: 1 in, 6 out]
        n194 = call-poly <instrlib>:"Configuration (Read).vi"("error in"=w427, "Mercury Reference In"=w426) -> ("error out"=w423:errorcluster, "Mode"=→"String":T48, "Mercury Reference Out"=w424:T42)  [unwired: 1 in, 6 out]
        n195 = Get Date/Time In Seconds() -> (seconds since 1Jan1904=w432:timestamp)
        n196 = call-poly <instrlib>:"Configuration (Set).vi"("error in"=w423, "time stamp"=w432, "Mercury Reference In"=w424) -> ("error out"=w417:errorcluster, "Response"=→"Set Date Response":T44)  [unwired: 1 in, 6 out]
        n197 = call <vilib>:"Add State(s) to Queue__JKI_lib_State_Machine.vi"("State(s) in (\"\")"=w457) -> ("States Out"=w456:string)  [unwired: 14 in]
      }
      frame "Mercury: Query ITC: Temperature" {
        # "Temperature"
        n198 = Unbundle By Name(w502) -> ("Mercury ITC Ref"=w459:T46)
        n199 = local read "ITC Devices"() -> (w458:string[])
        n200 = Index Array(array=w458, index=3) -> (element=w460:string)
        n201 = call-poly <instrlib>:"Open.vi"("error in (no error)"=w465, "Device Identifier"=w460, "Mercury Reference In"=w459) -> ("error out"=w477:errorcluster, "Mercury Reference Out"=w478:T42)  [unwired: 7 out]
        n202 = call-poly <instrlib>:"Configuration (Read).vi"("error in"=w477, "Mercury Reference In"=w478) -> ("error out"=w469:errorcluster, "Serial Number"=→"Temp S/N":string, "Mercury Reference Out"=w468:T42)  [unwired: 1 in, 6 out]
        n203 = call-poly <instrlib>:"Configuration (Read).vi"("error in"=w469, "Mercury Reference In"=w468) -> ("error out"=w471:errorcluster, "Nickname"=→"T Nickname":string, "Mercury Reference Out"=w470:T42)  [unwired: 1 in, 6 out]
        n204 = call-poly <instrlib>:"Configuration (Read).vi"("error in"=w471, "Mercury Reference In"=w470) -> ("error out"=w474:errorcluster, "Unit"=→"Unit":T2, "Excitation Magnitude"=→"Excitation Magnitude":dbl, "Mercury Reference Out"=w473:T42)  [unwired: 1 in, 5 out]
        n205 = call-poly <instrlib>:"Configuration (Read).vi"("error in"=w474, "Mercury Reference In"=w473) -> ("error out"=w463:errorcluster, "Sensor Type"=→"Sensor Type":T5, "Mercury Reference Out"=w461:T42)  [unwired: 1 in, 6 out]
        n206 = call-poly <instrlib>:"Configuration (Read).vi"("error in"=w463, "Mercury Reference In"=w461) -> ("error out"=w480:errorcluster, "Excitation Type"=→"Excitation Type":T7, "Mercury Reference Out"=w481:T42)  [unwired: 1 in, 6 out]
        n207 = call-poly <instrlib>:"Configuration (Read).vi"("error in"=w480, "Mercury Reference In"=w481) -> ("error out"=w482:errorcluster, "Unit"=→"H Unit":T2, "Hot Limit"=→"Hot Limit":dbl, "Mercury Reference Out"=w483:T42)  [unwired: 1 in, 5 out]
        n208 = call-poly <instrlib>:"Configuration (Read).vi"("error in"=w482, "Mercury Reference In"=w483) -> ("error out"=w489:errorcluster, "Unit"=→"C Unit":T2, "Cold Limit"=→"Cold Limit":dbl, "Mercury Reference Out"=w488:T42)  [unwired: 1 in, 5 out]
        n209 = call-poly <instrlib>:"Signals (Read).vi"("error in"=w489, "Mercury Reference In"=w488) -> ("error out"=w493:errorcluster, "Unit"=→"V Unit":T2, "Voltage"=→"Voltage":dbl, "Mercury Reference Out"=w492:T42)  [unwired: 1 in, 5 out]
        n210 = call-poly <instrlib>:"Signals (Read).vi"("error in"=w493, "Mercury Reference In"=w492) -> ("error out"=w494:errorcluster, "Unit"=→"T Unit":T2, "Temperature"=→"Temperature":dbl, "Mercury Reference Out"=w497:T42)  [unwired: 1 in, 5 out]
        n211 = call-poly <instrlib>:"Configuration (Read).vi"("error in"=w494, "Mercury Reference In"=w497) -> ("error out"=w500:errorcluster, "Device Details"=→"Temperature Device Settings":T3, "Mercury Reference Out"=w499:T42)  [unwired: 1 in, 6 out]
        n212 = call-poly <instrlib>:"Configuration (Read).vi"("error in"=w500, "Mercury Reference In"=w499) -> ("error out"=w464:errorcluster, "Loop Details"=→"T Loop Details":T10)  [unwired: 1 in, 7 out]
        n213 = call <vilib>:"Add State(s) to Queue__JKI_lib_State_Machine.vi"("State(s) in (\"\")"=w503) -> ("States Out"=w504:string)  [unwired: 14 in]
      }
      frame "Mercury: Query ITC: Heater" {
        # "Heater"
        n214 = Unbundle By Name(w509) -> ("Mercury ITC Ref"=w508:T46)
        n215 = local read "ITC Devices"() -> (w510:string[])
        n216 = Index Array(array=w510, index=2) -> (element=w505:string)
        n217 = call-poly <instrlib>:"Open.vi"("error in (no error)"=w512, "Device Identifier"=w505, "Mercury Reference In"=w508) -> ("error out"=w515:errorcluster, "Mercury Reference Out"=w514:T42)  [unwired: 7 out]
        n218 = call-poly <instrlib>:"Configuration (Read).vi"("error in"=w515, "Mercury Reference In"=w514) -> ("error out"=w522:errorcluster, "Device Details"=→"Heater Device Settings":T12, "Mercury Reference Out"=w521:T42)  [unwired: 1 in, 6 out]
        n219 = call-poly <instrlib>:"Configuration (Read).vi"("error in"=w522, "Mercury Reference In"=w521) -> ("error out"=w524:errorcluster, "Nickname"=→"Htr Nickname":string, "Mercury Reference Out"=w523:T42)  [unwired: 1 in, 6 out]
        n220 = call-poly <instrlib>:"Configuration (Read).vi"("error in"=w524, "Mercury Reference In"=w523) -> ("error out"=w517:errorcluster, "Serial Number"=→"Htr S/N":string, "Mercury Reference Out"=w516:T42)  [unwired: 1 in, 6 out]
        n221 = call-poly <instrlib>:"Configuration (Read).vi"("error in"=w517, "Mercury Reference In"=w516) -> ("error out"=w513:errorcluster, "Unit"=→"Volt Unit":T2, "Voltage Limit"=→"Htr Voltage Limit":dbl, "Mercury Reference Out"=w507:T42)  [unwired: 1 in, 5 out]
        n222 = call-poly <instrlib>:"Configuration (Read).vi"("error in"=w513, "Mercury Reference In"=w507) -> ("error out"=w527:errorcluster, "Unit"=→"Res Unit":T2, "Nominal Resistance"=→"Htr Resistance":dbl, "Mercury Reference Out"=w528:T42)  [unwired: 1 in, 5 out]
        n223 = call-poly <instrlib>:"Configuration (Read).vi"("error in"=w527, "Mercury Reference In"=w528) -> ("error out"=w534:errorcluster, "Unit"=→"Power Unit":T2, "Maximum Power"=→"Maximum Power":dbl, "Mercury Reference Out"=w533:T42)  [unwired: 1 in, 5 out]
        n224 = call-poly <instrlib>:"Signals (Read).vi"("error in"=w534, "Mercury Reference In"=w533) -> ("error out"=w536:errorcluster, "Unit"=→"Htr V Unit":T2, "Voltage"=→"Htr Voltage":dbl, "Mercury Reference Out"=w535:T42)  [unwired: 1 in, 5 out]
        n225 = call-poly <instrlib>:"Signals (Read).vi"("error in"=w536, "Mercury Reference In"=w535) -> ("error out"=w538:errorcluster, "Unit"=→"Htr P Unit":T2, "Power"=→"Htr Power":dbl, "Mercury Reference Out"=w537:T42)  [unwired: 1 in, 5 out]
        n226 = call-poly <instrlib>:"Signals (Read).vi"("error in"=w538, "Mercury Reference In"=w537) -> ("error out"=w506:errorcluster, "Unit"=→"Htr C Unit":T2, "Current"=→"Htr Current":dbl)  [unwired: 1 in, 6 out]
        n227 = call <vilib>:"Add State(s) to Queue__JKI_lib_State_Machine.vi"("State(s) in (\"\")"=w545) -> ("States Out"=w546:string)  [unwired: 14 in]
      }
      frame "Mercury: Query ITC: Aux" {
        # "Auxiliary"
        n228 = Unbundle By Name(w552) -> ("Mercury ITC Ref"=w547:T46)
        n229 = local read "ITC Devices"() -> (w550:string[])
        n230 = Index Array(array=w550, index=0) -> (element=w548:string)
        n231 = call-poly <instrlib>:"Open.vi"("error in (no error)"=w554, "Device Identifier"=w548, "Mercury Reference In"=w547) -> ("error out"=w574:errorcluster, "Mercury Reference Out"=w575:T42)  [unwired: 7 out]
        n232 = call-poly <instrlib>:"Configuration (Read).vi"("error in"=w574, "Mercury Reference In"=w575) -> ("error out"=w578:errorcluster, "Auxiliary Device Details"=→"Auxiliary Device Details":T20, "Mercury Reference Out"=w577:T42)  [unwired: 1 in, 6 out]
        n233 = call-poly <instrlib>:"Configuration (Read).vi"("error in"=w578, "Mercury Reference In"=w577) -> ("error out"=w581:errorcluster, "Serial Number"=→"Aux S/N":string, "Mercury Reference Out"=w580:T42)  [unwired: 1 in, 6 out]
        n234 = call-poly <instrlib>:"Configuration (Read).vi"("error in"=w581, "Mercury Reference In"=w580) -> ("error out"=w583:errorcluster, "Unit"=→"Unit 2":T2, "Min Flow"=→"Min Flow":dbl, "Mercury Reference Out"=w582:T42)  [unwired: 1 in, 5 out]
        n235 = call-poly <instrlib>:"Configuration (Read).vi"("error in"=w583, "Mercury Reference In"=w582) -> ("error out"=w585:errorcluster, "Unit"=→"Unit 3":T2, "Scaling Factor"=→"Scaling Factor":dbl, "Mercury Reference Out"=w584:T42)  [unwired: 1 in, 5 out]
        n236 = call-poly <instrlib>:"Configuration (Read).vi"("error in"=w585, "Mercury Reference In"=w584) -> ("error out"=w553:errorcluster, "Unit"=→"Unit 4":T2, "Temp Err"=→"Temp Err":dbl, "Mercury Reference Out"=w549:T42)  [unwired: 1 in, 5 out]
        n237 = call-poly <instrlib>:"Configuration (Read).vi"("error in"=w553, "Mercury Reference In"=w549) -> ("error out"=w557:errorcluster, "Unit"=→"Unit 5":T2, "Temp V Err"=→"Temp V Err":dbl, "Mercury Reference Out"=w556:T42)  [unwired: 1 in, 5 out]
        n238 = call-poly <instrlib>:"Configuration (Read).vi"("error in"=w557, "Mercury Reference In"=w556) -> ("error out"=w559:errorcluster, "Unit"=→"Unit 6":T2, "Gear"=→"Gear":u32, "Mercury Reference Out"=w558:T42)  [unwired: 1 in, 5 out]
        n239 = call-poly <instrlib>:"Configuration (Read).vi"("error in"=w559, "Mercury Reference In"=w558) -> ("error out"=w567:errorcluster, "Unit"=→"Unit 7":T2, "Speed"=→"Speed":u32, "Mercury Reference Out"=w566:T42)  [unwired: 1 in, 5 out]
        n240 = call-poly <instrlib>:"Signals (Read).vi"("error in"=w567, "Mercury Reference In"=w566) -> ("error out"=w569:errorcluster, "Unit"=→"Unit":T2, "Position"=→"Position":u32, "Mercury Reference Out"=w568:T42)  [unwired: 1 in, 5 out]
        n241 = call-poly <instrlib>:"Signals (Read).vi"("error in"=w569, "Mercury Reference In"=w568) -> ("error out"=w555:errorcluster, "Unit"=→"Unit":T2, "% Open"=→"% Open":dbl)  [unwired: 1 in, 6 out]
        n242 = call <vilib>:"Add State(s) to Queue__JKI_lib_State_Machine.vi"("State(s) in (\"\")"=w592) -> ("States Out"=w593:string)  [unwired: 14 in]
      }
      frame "Mercury: Query ITC: Pressure" {
        # "Pressure"
        n243 = Unbundle By Name(w599) -> ("Mercury ITC Ref"=w596:T46)
        n244 = local read "ITC Devices"() -> (w598:string[])
        n245 = Index Array(array=w598, index=1) -> (element=w595:string)
        n246 = call-poly <instrlib>:"Open.vi"("error in (no error)"=w594, "Device Identifier"=w595, "Mercury Reference In"=w596) -> ("error out"=w602:errorcluster, "Mercury Reference Out"=w603:T42)  [unwired: 7 out]
        n247 = call-poly <instrlib>:"Configuration (Read).vi"("error in"=w602, "Mercury Reference In"=w603) -> ("error out"=w604:errorcluster, "Device Details"=→"Pressure Device":T14, "Mercury Reference Out"=w605:T42)  [unwired: 1 in, 6 out]
        n248 = call-poly <instrlib>:"Configuration (Read).vi"("error in"=w604, "Mercury Reference In"=w605) -> ("error out"=w609:errorcluster, "Nickname"=→"Nickname":string, "Mercury Reference Out"=w610:T42)  [unwired: 1 in, 6 out]
        n249 = call-poly <instrlib>:"Signals (Read).vi"("error in"=w609, "Mercury Reference In"=w610) -> ("error out"=w607:errorcluster, "Current"=→"Current":dbl, "Mercury Reference Out"=w608:T42)  [unwired: 1 in, 6 out]
        n250 = call-poly <instrlib>:"Signals (Read).vi"("error in"=w607, "Mercury Reference In"=w608) -> ("error out"=w600:errorcluster, "Voltage"=→"Voltage":dbl)  [unwired: 1 in, 7 out]
        n251 = call <vilib>:"Add State(s) to Queue__JKI_lib_State_Machine.vi"("State(s) in (\"\")"=w613) -> ("States Out"=w614:string)  [unwired: 14 in]
      }
      frame "Mercury: Query IPS: System" {
        # "Your code here.\n(You can make a copy of, or modify, this frame)"
        n252 = Unbundle By Name(w656) -> ("Mercury IPS Ref"=w617:T42)
        n253 = call-poly <instrlib>:"Configuration (Read).vi"("error in"=w622, "Mercury Reference In"=w617) -> ("error out"=w642:errorcluster, "Devices"=→"IPS Devices":string[], "Mercury Reference Out"=w641:T42)  [unwired: 1 in, 6 out]
        n254 = call-poly <instrlib>:"Configuration (Read).vi"("error in"=w642, "Mercury Reference In"=w641) -> ("error out"=w646:errorcluster, "Automatic Dimming"=→"Automatic Dimming 2":string, "Mercury Reference Out"=w645:T42)  [unwired: 1 in, 6 out]
        n255 = call-poly <instrlib>:"Configuration (Read).vi"("error in"=w646, "Mercury Reference In"=w645) -> ("error out"=w643:errorcluster, "Dimming Time"=→"Dimming Time 2":string, "Mercury Reference Out"=w644:T42)  [unwired: 1 in, 6 out]
        n256 = call-poly <instrlib>:"Configuration (Read).vi"("error in"=w643, "Mercury Reference In"=w644) -> ("error out"=w640:errorcluster, "Display Brightness"=→"Display Brightness 2":string, "Mercury Reference Out"=w639:T42)  [unwired: 1 in, 6 out]
        n257 = call-poly <instrlib>:"Configuration (Read).vi"("error in"=w640, "Mercury Reference In"=w639) -> ("error out"=w649:errorcluster, "Date"=→"Date 2":string, "Mercury Reference Out"=w650:T42)  [unwired: 1 in, 6 out]
        n258 = call-poly <instrlib>:"Configuration (Read).vi"("error in"=w649, "Mercury Reference In"=w650) -> ("error out"=w647:errorcluster, "Time"=→"Time 2":string, "Mercury Reference Out"=w648:T42)  [unwired: 1 in, 6 out]
        n259 = call-poly <instrlib>:"Configuration (Read).vi"("error in"=w647, "Mercury Reference In"=w648) -> ("error out"=w621:errorcluster, "time stamp"=→"time stamp 2":timestamp, "Mercury Reference Out"=w618:T42)  [unwired: 1 in, 6 out]
        n260 = call-poly <instrlib>:"Configuration (Read).vi"("error in"=w621, "Mercury Reference In"=w618) -> ("error out"=w623:errorcluster, "Hardware Version"=→"Hardware Version 2":string, "Mercury Reference Out"=w624:T42)  [unwired: 1 in, 6 out]
        n261 = call-poly <instrlib>:"Configuration (Read).vi"("error in"=w623, "Mercury Reference In"=w624) -> ("error out"=w625:errorcluster, "Firmware Version"=→"Firmware Version 2":string, "Mercury Reference Out"=w626:T42)  [unwired: 1 in, 6 out]
        n262 = call-poly <instrlib>:"Configuration (Read).vi"("error in"=w625, "Mercury Reference In"=w626) -> ("error out"=w631:errorcluster, "Serial Number"=→"Serial Number 2":string, "Mercury Reference Out"=w632:T42)  [unwired: 1 in, 6 out]
        n263 = call-poly <instrlib>:"Configuration (Read).vi"("error in"=w631, "Mercury Reference In"=w632) -> ("error out"=w627:errorcluster, "Free Space"=→"Free Space 2":i32, "Mercury Reference Out"=w628:T42)  [unwired: 1 in, 6 out]
        n264 = call-poly <instrlib>:"Configuration (Read).vi"("error in"=w627, "Mercury Reference In"=w628) -> ("error out"=w630:errorcluster, "Mode"=→"String 2":T48, "Mercury Reference Out"=w629:T42)  [unwired: 1 in, 6 out]
        n265 = Get Date/Time In Seconds() -> (seconds since 1Jan1904=w638:timestamp)
        n266 = call-poly <instrlib>:"Configuration (Set).vi"("error in"=w630, "time stamp"=w638, "Mercury Reference In"=w629) -> ("error out"=w620:errorcluster, "Response"=→"Set Date Response 2":T44)  [unwired: 1 in, 6 out]
        n267 = call <vilib>:"Add State(s) to Queue__JKI_lib_State_Machine.vi"("State(s) in (\"\")"=w658) -> ("States Out"=w657:string)  [unwired: 14 in]
      }
      frame "Mercury: Query IPS: LVL" {
        # "Level"
        n268 = Unbundle By Name(w698) -> ("Mercury IPS Ref"=w661:T42)
        n269 = local read "IPS Devices"() -> (w697:string[])
        n270 = Index Array(array=w697, index=0) -> (element=w660:string)
        n271 = call-poly <instrlib>:"Open.vi"("error in (no error)"=w667, "Device Identifier"=w660, "Mercury Reference In"=w661) -> ("error out"=w683:errorcluster, "Mercury Reference Out"=w682:T42)  [unwired: 7 out]
        n272 = call-poly <instrlib>:"Configuration (Read).vi"("error in"=w683, "Mercury Reference In"=w682) -> ("error out"=w688:errorcluster, "LVL Device Settings"=→"LVL Device DetailSettings":T22, "Mercury Reference Out"=w685:T42)  [unwired: 1 in, 6 out]
        n273 = call-poly <instrlib>:"Configuration (Read).vi"("error in"=w688, "Mercury Reference In"=w685) -> ("error out"=w689:errorcluster, "Serial Number"=→"LVL S/N":string, "Mercury Reference Out"=w687:T42)  [unwired: 1 in, 6 out]
        n274 = call-poly <instrlib>:"Configuration (Read).vi"("error in"=w689, "Mercury Reference In"=w687) -> ("error out"=w692:errorcluster, "Resistance Configuration"=→"He Res Config":T27, "Mercury Reference Out"=w691:T42)  [unwired: 1 in, 6 out]
        n275 = call-poly <instrlib>:"Configuration (Read).vi"("error in"=w692, "Mercury Reference In"=w691) -> ("error out"=w694:errorcluster, "Magnitude"=→"LVL P Magnitude":dbl, "Mercury Reference Out"=w693:T42)  [unwired: 1 in, 6 out]
        n276 = call-poly <instrlib>:"Configuration (Read).vi"("error in"=w694, "Mercury Reference In"=w693) -> ("error out"=w666:errorcluster, "Duration"=→"LVL P Duration":dbl, "Mercury Reference Out"=w664:T42)  [unwired: 1 in, 6 out]
        n277 = call-poly <instrlib>:"Configuration (Read).vi"("error in"=w666, "Mercury Reference In"=w664) -> ("error out"=w670:errorcluster, "Freq 100%"=→"N Freq 100%":dbl, "Mercury Reference Out"=w669:T42)  [unwired: 1 in, 6 out]
        n278 = call-poly <instrlib>:"Configuration (Read).vi"("error in"=w670, "Mercury Reference In"=w669) -> ("error out"=w673:errorcluster, "Pulse Period"=→"N Pulse Period":dbl, "Mercury Reference Out"=w672:T42)  [unwired: 1 in, 6 out]
        n279 = call-poly <instrlib>:"Signals (Read).vi"("error in"=w673, "Mercury Reference In"=w672) -> ("error out"=w675:errorcluster, "Resistance"=→"He Resistance":dbl, "Mercury Reference Out"=w674:T42)  [unwired: 1 in, 6 out]
        n280 = call-poly <instrlib>:"Signals (Read).vi"("error in"=w675, "Mercury Reference In"=w674) -> ("error out"=w677:errorcluster, "Level"=→"He Level" →"He LEVEL":dbl, "Mercury Reference Out"=w676:T42)  [unwired: 1 in, 6 out]
        n281 = call-poly <instrlib>:"Signals (Read).vi"("error in"=w677, "Mercury Reference In"=w676) -> ("error out"=w679:errorcluster, "Counter"=→"N Counter":u32, "Mercury Reference Out"=w678:T42)  [unwired: 1 in, 6 out]
        n282 = call-poly <instrlib>:"Signals (Read).vi"("error in"=w679, "Mercury Reference In"=w678) -> ("error out"=w665:errorcluster, "Level"=→"N Level" →"N2 LEVEL":dbl)  [unwired: 1 in, 7 out]
        n283 = call <vilib>:"Add State(s) to Queue__JKI_lib_State_Machine.vi"("State(s) in (\"\")"=w699) -> ("States Out"=w700:string)  [unwired: 14 in]
      }
      frame "Mercury: Query IPS: Temperature" {
        n284 = Unbundle By Name(w745) -> ("Mercury IPS Ref"=w702:T42)
        n285 = local read "IPS Devices"() -> (w744:string[])
        n286 = Index Array(array=w744, index=4) -> (element=w703:string)
        n287 = call-poly <instrlib>:"Open.vi"("error in (no error)"=w701, "Device Identifier"=w703, "Mercury Reference In"=w702) -> ("error out"=w732:errorcluster, "Mercury Reference Out"=w727:T42)  [unwired: 7 out]
        n288 = call-poly <instrlib>:"Configuration (Read).vi"("error in"=w732, "Mercury Reference In"=w727) -> ("error out"=w733:errorcluster, "Serial Number"=→"Temp S/N 2":string, "Mercury Reference Out"=w728:T42)  [unwired: 1 in, 6 out]
        n289 = call-poly <instrlib>:"Configuration (Read).vi"("error in"=w733, "Mercury Reference In"=w728) -> ("error out"=w734:errorcluster, "Nickname"=→"T Nickname 2":string, "Mercury Reference Out"=w729:T42)  [unwired: 1 in, 6 out]
        n290 = call-poly <instrlib>:"Configuration (Read).vi"("error in"=w734, "Mercury Reference In"=w729) -> ("error out"=w735:errorcluster, "Unit"=→"Unit 12":T2, "Excitation Magnitude"=→"Excitation Magnitude 2":dbl, "Mercury Reference Out"=w730:T42)  [unwired: 1 in, 5 out]
        n291 = call-poly <instrlib>:"Configuration (Read).vi"("error in"=w735, "Mercury Reference In"=w730) -> ("error out"=w736:errorcluster, "Sensor Type"=→"Sensor Type 2":T5, "Mercury Reference Out"=w731:T42)  [unwired: 1 in, 6 out]
        n292 = call-poly <instrlib>:"Configuration (Read).vi"("error in"=w736, "Mercury Reference In"=w731) -> ("error out"=w706:errorcluster, "Excitation Type"=→"Excitation Type 2":T7, "Mercury Reference Out"=w705:T42)  [unwired: 1 in, 6 out]
        n293 = call-poly <instrlib>:"Configuration (Read).vi"("error in"=w706, "Mercury Reference In"=w705) -> ("error out"=w712:errorcluster, "Unit"=→"H Unit 2":T2, "Hot Limit"=→"Hot Limit 2":dbl, "Mercury Reference Out"=w707:T42)  [unwired: 1 in, 5 out]
        n294 = call-poly <instrlib>:"Configuration (Read).vi"("error in"=w712, "Mercury Reference In"=w707) -> ("error out"=w713:errorcluster, "Unit"=→"C Unit 2":T2, "Cold Limit"=→"Cold Limit 2":dbl, "Mercury Reference Out"=w708:T42)  [unwired: 1 in, 5 out]
        n295 = call-poly <instrlib>:"Signals (Read).vi"("error in"=w713, "Mercury Reference In"=w708) -> ("error out"=w714:errorcluster, "Unit"=→"V Unit 2":T2, "Voltage"=→"Voltage 2":dbl, "Mercury Reference Out"=w709:T42)  [unwired: 1 in, 5 out]
        n296 = call-poly <instrlib>:"Signals (Read).vi"("error in"=w714, "Mercury Reference In"=w709) -> ("error out"=w715:errorcluster, "Unit"=→"T Unit 2":T2, "Temperature"=→"Temperature 2":dbl, "Mercury Reference Out"=w710:T42)  [unwired: 1 in, 5 out]
        n297 = call-poly <instrlib>:"Configuration (Read).vi"("error in"=w715, "Mercury Reference In"=w710) -> ("error out"=w716:errorcluster, "Device Details"=→"Temperature Device Settings 2":T3, "Mercury Reference Out"=w711:T42)  [unwired: 1 in, 6 out]
        n298 = call-poly <instrlib>:"Configuration (Read).vi"("error in"=w716, "Mercury Reference In"=w711) -> ("error out"=w704:errorcluster, "Loop Details"=→"T Loop Details 2":T10)  [unwired: 1 in, 7 out]
        n299 = call <vilib>:"Add State(s) to Queue__JKI_lib_State_Machine.vi"("State(s) in (\"\")"=w746) -> ("States Out"=w747:string)  [unwired: 14 in]
      }
      frame "Mercury: Query IPS: Magnet" {
        n300 = Unbundle By Name(w786) -> ("Mercury IPS Ref"=w752:T42)
        n301 = call-poly <instrlib>:"Open.vi"("error in (no error)"=w748, "Device Identifier"="Device Identifier", "Mercury Reference In"=w752) -> ("error out"=w771:errorcluster, "Mercury Reference Out"=w770:T42)  [unwired: 7 out]
        n302 = call-poly <instrlib>:"Configuration (Read).vi"("error in"=w771, "Mercury Reference In"=w770) -> ("error out"=w774:errorcluster, "Magnet Device Details"=→"Magnet Device Details":T30, "Mercury Reference Out"=w773:T42)  [unwired: 1 in, 6 out]
        n303 = call-poly <instrlib>:"Configuration (Read).vi"("error in"=w774, "Mercury Reference In"=w773) -> ("error out"=w777:errorcluster, "Serial Number"=→"Mag S/N":string, "Mercury Reference Out"=w776:T42)  [unwired: 1 in, 6 out]
        n304 = call-poly <instrlib>:"Configuration (Read).vi"("error in"=w777, "Mercury Reference In"=w776) -> ("error out"=w780:errorcluster, "Bipolar Output"=→"Bipolar Output":string, "Mercury Reference Out"=w779:T42)  [unwired: 1 in, 6 out]
        n305 = call-poly <instrlib>:"Configuration (Read).vi"("error in"=w780, "Mercury Reference In"=w779) -> ("error out"=w783:errorcluster, "Out Config"=→"Out Config":T49, "Mercury Reference Out"=w782:T42)  [unwired: 1 in, 6 out]
        n306 = call-poly <instrlib>:"Configuration (Read).vi"("error in"=w783, "Mercury Reference In"=w782) -> ("error out"=w754:errorcluster, "Unit"=→"Unit 8":T2, "Current Limit"=→"Current Limit":dbl, "Mercury Reference Out"=w751:T42)  [unwired: 1 in, 5 out]
        n307 = call-poly <instrlib>:"Configuration (Read).vi"("error in"=w754, "Mercury Reference In"=w751) -> ("error out"=w757:errorcluster, "Unit"=→"Unit 9":T2, "AtoB"=→"AtoB":dbl, "Mercury Reference Out"=w756:T42)  [unwired: 1 in, 5 out]
        n308 = call-poly <instrlib>:"Configuration (Read).vi"("error in"=w757, "Mercury Reference In"=w756) -> ("error out"=w760:errorcluster, "Switch Present"=→"Switch Present":string, "Mercury Reference Out"=w759:T42)  [unwired: 1 in, 6 out]
        n309 = call-poly <instrlib>:"Configuration (Read).vi"("error in"=w760, "Mercury Reference In"=w759) -> ("error out"=w765:errorcluster, "Unit"=→"Unit 10":T2, "SW VLIM"=→"SW VLIM":dbl, "Mercury Reference Out"=w764:T42)  [unwired: 1 in, 5 out]
        n310 = call-poly <instrlib>:"Signals (Read).vi"("error in"=w765, "Mercury Reference In"=w764) -> ("error out"=w767:errorcluster, "Unit"=→"Unit 11":T2, "Current Rate"=→"Current Rate":dbl, "Mercury Reference Out"=w766:T42)  [unwired: 1 in, 5 out]
        n311 = call-poly <instrlib>:"Signals (Read).vi"("error in"=w767, "Mercury Reference In"=w766) -> ("error out"=w753:errorcluster, "PSU Act Stat"=→"PSU Act Stat":T34)  [unwired: 1 in, 7 out]
        n312 = call <vilib>:"Add State(s) to Queue__JKI_lib_State_Machine.vi"("State(s) in (\"\")"=w787) -> ("States Out"=w788:string)  [unwired: 14 in]
      }
      frame "Mercury: IPS: Idle - 1" {
        n313 = Unbundle By Name(w823) -> ("Mercury IPS Ref"=w790:T42)
        n314 = local read "Device Identifier"() -> (w803:T32)
        n315 = call-poly <instrlib>:"Configuration (Read).vi"("error in"=w822, "Mercury Reference In"=w790) -> ("error out"=w810:errorcluster, "Time"=w815:string, "Mercury Reference Out"=w811:T42)  [unwired: 1 in, 6 out]
        n316 = local write "Time 2"(w815) -> ()
        n317 = call-poly <instrlib>:"Open.vi"("error in (no error)"=w810, "Device Identifier"=w803, "Mercury Reference In"=w811) -> ("error out"=w809:errorcluster, "Mercury Reference Out"=w808:T42)  [unwired: 7 out]
        n318 = call-poly <instrlib>:"Signals (Read).vi"("error in"=w809, "Mercury Reference In"=w808) -> ("error out"=w821:errorcluster, "Switch Heater Status"=w812:string, "Mercury Reference Out"=w818:T42)  [unwired: 1 in, 6 out]
        n319 = Equal?(x=w812, y="ON") -> (x = y?=→"SWITCH HEATER":bool)
        n320 = call-poly <instrlib>:"Signals (Read).vi"("error in"=w821, "Mercury Reference In"=w818) -> ("error out"=w820:errorcluster, "Current"=→"Current (A)" →"Current (A)":dbl, "Mercury Reference Out"=w817:T42)  [unwired: 1 in, 6 out]
        n321 = call-poly <instrlib>:"Signals (Read).vi"("error in"=w820, "Mercury Reference In"=w817) -> ("error out"=w802:errorcluster, "Voltage"=→"Voltage (V)" →"Voltage (V)":dbl, "Mercury Reference Out"=w801:T42)  [unwired: 1 in, 6 out]
        n322 = call-poly <instrlib>:"Signals (Read).vi"("error in"=w802, "Mercury Reference In"=w801) -> ("error out"=w804:errorcluster, "Field"=→"Power Supply Field (T)":dbl, "Mercury Reference Out"=w807:T42)  [unwired: 1 in, 6 out]
        n323 = call-poly <instrlib>:"Signals (Read).vi"("error in"=w804, "Mercury Reference In"=w807) -> ("error out"=w805:errorcluster, "Target Field Rate"=→"Target Field Rate (T/min)":dbl, "Mercury Reference Out"=w806:T42)  [unwired: 1 in, 6 out]
        n324 = call-poly <instrlib>:"Signals (Read).vi"("error in"=w805, "Mercury Reference In"=w806) -> ("error out"=w800:errorcluster, "Target Field"=→"Target Field (T)":dbl, "Mercury Reference Out"=w799:T42)  [unwired: 1 in, 6 out]
        n325 = call-poly <instrlib>:"Signals (Read).vi"("error in"=w800, "Mercury Reference In"=w799) -> ("error out"=w819:errorcluster, "Persistant Field"=→"Magnet Field (T)" →"Magnet Field (T)":dbl, "Mercury Reference Out"=w816:T42)  [unwired: 1 in, 6 out]
        n326 = call-poly <instrlib>:"Signals (Read).vi"("error in"=w819, "Mercury Reference In"=w816) -> ("error out"=w789:errorcluster, "PSU Act Stat"=w791:T34)  [unwired: 1 in, 7 out]
        n327 = local write "PSU Act Stat"(w791) -> ()
        n328 = case shown="\"CLMP\"" w791 {
          selector: w791 -> [w826 _ _ _ _]
          tunnel: [w826 "Holding" "Ramping to Setpoint" "Ramping to Zero" "Clamped"] -> w798
          frame Default {
          }
          frame "HOLD" {
          }
          frame "RTOS" {
          }
          frame "RTOZ" {
          }
          frame "CLMP" {
          }
        }
        "Magnet Status" <- w798
        n329 = call <vilib>:"Add State(s) to Queue__JKI_lib_State_Machine.vi"("State(s) in (\"\")"=w824) -> ("States Out"=w825:string)  [unwired: 14 in]
      }
      frame "Mercury: IPS: Idle - 2" {
        n330 = Unbundle By Name(w877) -> ("Mercury IPS Ref"=w832:T42)
        n331 = local read "IPS Devices"() -> (w871:string[])
        n332 = Index Array(array=w871, index=0) -> (element=w870:string)
        n333 = call-poly <instrlib>:"Open.vi"("error in (no error)"=w855, "Device Identifier"=w870, "Mercury Reference In"=w832) -> ("error out"=w873:errorcluster, "Mercury Reference Out"=w874:T42)  [unwired: 7 out]
        n334 = call-poly <instrlib>:"Signals (Read).vi"("error in"=w873, "Mercury Reference In"=w874) -> ("error out"=w875:errorcluster, "Level"=w834:dbl, "Mercury Reference Out"=w876:T42)  [unwired: 1 in, 6 out]
        "He LVL Chart" <- w834
        n335 = Greater?(x=w834, y=20.0) -> (0:w852:bool)
        n336 = Greater?(x=w834, y=50.0) -> (0:w853:bool)
        n337 = call-poly <instrlib>:"Signals (Read).vi"("error in"=w875, "Mercury Reference In"=w876) -> ("error out"=w860:errorcluster, "Level"=w833:dbl)  [unwired: 1 in, 7 out]
        "N2 LVL Chart" <- w833
        n338 = case shown="False" w852 {
          tunnel: [w885 u32 6618880] -> w842
          tunnel: w853 -> [w886 _]
          frame False {
            n339 = case shown="True" w886 {
              tunnel: [u32 16711680 u32 16776704] -> w885
              frame False {
              }
              frame True {
              }
            }
          }
          frame True {
          }
        }
        n340 = local write "He LEVEL"(w834) -> ()
        n341 = local read "IPS Devices"() -> (w865:string[])
        n342 = property on="He LVL Chart" class="Slide (strict)"("Fill Color"=w842) -> ()  [unwired: 2 in, 2 out]
        n343 = local write "N2 LEVEL"(w833) -> ()
        n344 = Index Array(array=w865, index=4) -> (element=w863:string)
        n345 = local read "Target Field Rate (T/min)"() -> (w847:dbl)
        n346 = local read "Power Supply Field (T)"() -> (w850:dbl)
        n347 = call-poly <instrlib>:"Open.vi"("error in (no error)"=w860, "Device Identifier"=w863, "Mercury Reference In"=w832) -> ("error out"=w862:errorcluster, "Mercury Reference Out"=w861:T42)  [unwired: 7 out]
        n348 = local read "Magnet Field (T)"() -> (w849:dbl)
        n349 = local read "Target Field (T)"() -> (w848:dbl)
        n350 = Greater?(x=w833, y=20.0) -> (0:w837:bool)
        n351 = Greater?(x=w833, y=50.0) -> (0:w836:bool)
        n352 = local read "Voltage (V)"() -> (w846:dbl)
        n353 = local read "Current (A)"() -> (w845:dbl)
        n354 = case shown="False" w837 {
          tunnel: [w880 u32 6618880] -> w835
          tunnel: w836 -> [w881 _]
          frame False {
            n355 = case shown="True" w881 {
              tunnel: [u32 16711680 u32 16776704] -> w880
              frame False {
              }
              frame True {
              }
            }
          }
          frame True {
          }
        }
        n356 = call-poly <instrlib>:"Signals (Read).vi"("error in"=w862, "Mercury Reference In"=w861) -> ("error out"=w858:errorcluster, "Temperature"=w856:dbl)  [unwired: 1 in, 7 out]
        "Magnet Temperature" <- w856
        n357 = property on="N2 LVL Chart" class="Slide (strict)"("Fill Color"=w835) -> ()  [unwired: 2 in, 2 out]
        n358 = Bundle(cluster=T39 {"Persistant Field"=0.0, "Field"=0.0, "Target Field"=0.0, "Target Field Rate"=0.0, "Voltage"=0.0, "Current"=0.0}, "Persistant Field"=w849, "Field"=w850, "Target Field"=w848, "Target Field Rate"=w847, "Voltage"=w846, "Current"=w845) -> (w844:T39)
        n359 = local read "PSU Act Stat"() -> (w843:string)
        n360 = Cluster To Array(cluster=w844) -> (array=w867:dbl[])
        n361 = call "FGV - Mercury Status.vi"("error in"=w858, "Function"=enum16{"write", "read"}."write", "satus"=w844) -> ("error out"=w857:errorcluster)  [unwired: 3 in, 1 out]
        n362 = property on="N2 LVL Chart" class="Slide (strict)"("Scale.Flipped"=FALSE) -> ()  [unwired: 2 in, 2 out]
        n363 = call "FGV - Mercury Action Status.vi"("error in"=w857, "Function"=enum16{"write", "read"}."write", "Mercury Status"=w843) -> ("error out"=w854:errorcluster)  [unwired: 3 in, 1 out]
        n364 = Build Array (concatenate)(w867, w833, w834, w856) -> (w866:dbl[])
        n365 = Build Array(w843) -> (w859:string[])
        n366 = call "1820_IPS_to_DSC.vi"("str"=w859, "dbl"=w866) -> ()  [unwired: 2 in]
        n367 = call <vilib>:"Add State(s) to Queue__JKI_lib_State_Machine.vi"("State(s) in (\"\")"=w878) -> ("States Out"=w879:string)  [unwired: 14 in]
      }
      frame "Mercury: ITC: Idle" {
        n368 = Unbundle By Name(w916) -> ("Mercury ITC Ref"=w896:T46)
        n369 = local read "ITC Devices"() -> (w912:string[])
        n370 = Index Array(array=w912, index=3) -> (element=w911:string)
        n371 = call-poly <instrlib>:"Open.vi"("error in (no error)"=w891, "Device Identifier"=w911, "Mercury Reference In"=w896) -> ("error out"=w910:errorcluster, "Mercury Reference Out"=w903:T42)  [unwired: 7 out]
        n372 = call-poly <instrlib>:"Signals (Read).vi"("error in"=w910, "Mercury Reference In"=w903) -> ("error out"=w909:errorcluster, "Temperature"=w894:dbl)  [unwired: 1 in, 7 out]
        "LPF Temperature" <- w894
        n373 = local read "ITC Devices"() -> (w915:string[])
        n374 = Index Array(array=w915, index=1) -> (element=w913:string)
        n375 = call-poly <instrlib>:"Open.vi"("error in (no error)"=w909, "Device Identifier"=w913, "Mercury Reference In"=w896) -> ("error out"=w908:errorcluster, "Mercury Reference Out"=w907:T42)  [unwired: 7 out]
        n376 = call-poly <instrlib>:"Configuration (Read).vi"("error in"=w908, "Mercury Reference In"=w907) -> ("error out"=w902:errorcluster, "Device Details"=w906:T14)  [unwired: 1 in, 7 out]
        n377 = local read "ITC Devices"() -> (w900:string[])
        n378 = Unbundle By Name(w906) -> ("Pressure Signals.Pressure"=w905:string)
        n379 = Index Array(array=w900, index=0) -> (element=w899:string)
        n380 = call-poly <instrlib>:"Open.vi"("error in (no error)"=w902, "Device Identifier"=w899, "Mercury Reference In"=w896) -> ("error out"=w898:errorcluster, "Mercury Reference Out"=w897:T42)  [unwired: 7 out]
        n381 = Fract/Exp String To Number(string=w905) -> (number=w893:dbl)  [unwired: 3 in, 1 out]
        "LPF Pressure" <- w893
        n382 = call-poly <instrlib>:"Signals (Read).vi"("error in"=w898, "Mercury Reference In"=w897) -> ("error out"=w890:errorcluster, "% Open"=w892:dbl)  [unwired: 1 in, 7 out]
        "LPF Needle Valve (%)" <- w892
        n383 = Build Array(w894, w893, w892) -> (w895:dbl[])
        n384 = call "1820_ITC_to_DSC.vi"("dbl"=w895) -> ()  [unwired: 3 in]
        n385 = call <vilib>:"Add State(s) to Queue__JKI_lib_State_Machine.vi"("State(s) in (\"\")"=w917) -> ("States Out"=w918:string)  [unwired: 14 in]
      }
      frame "Mercury: Empty" {
        n386 = Unbundle By Name(w920) -> ()  [unwired: 1 out]
        n387 = call <vilib>:"Add State(s) to Queue__JKI_lib_State_Machine.vi"("State(s) in (\"\")"=w921) -> ("States Out"=w922:string)  [unwired: 14 in]
      }
    }
  }
  n388 = disable-structure shown="Disabled" {
    frame Disabled {
      (unwired) FALSE
      n389 = call-poly <instrlib>:"Configuration (Read).vi"() -> ()  [unwired: 3 in, 9 out]
      n390 = local read "PS Heat"() -> ()  [unwired: 1 in]
      n391 = local read "Lambda"() -> ()  [unwired: 1 in]
    }
    frame Enabled {
    }
  }
